vi "Daj Boze nesto.vi"() -> ()   [LabVIEW 2014]
uses:
  Timer 2013/Control Timer.ctl
  <vilib>/ptbypt/NI_PtbyPt.lvlib
panel:
  in  "Emergency offAct":bool=TRUE
  in  "RightAct":bool
  in  "CenterAct":bool
  in  "LeftAct":bool
  in  "OffAct":bool=TRUE
  in  "OnAct":bool
  out "PumpFlag":bool
  out "SDFlag":bool
  out "error out":errorcluster
  in  "error in (no error)":errorcluster
  in  "Center":bool
  in  "Left":bool
  in  "Right":bool
  in  "Emergency off":bool=TRUE
  in  "Off":bool=TRUE
  in  "On":bool
  out "Stanje":string
  out "RightLED":bool
  out "LeftLED":bool
  out "CenterLED":bool
  out "Fault":bool
  out "On/Off":bool
  out "BrojacGreska":dbl
  out "Brojac":dbl
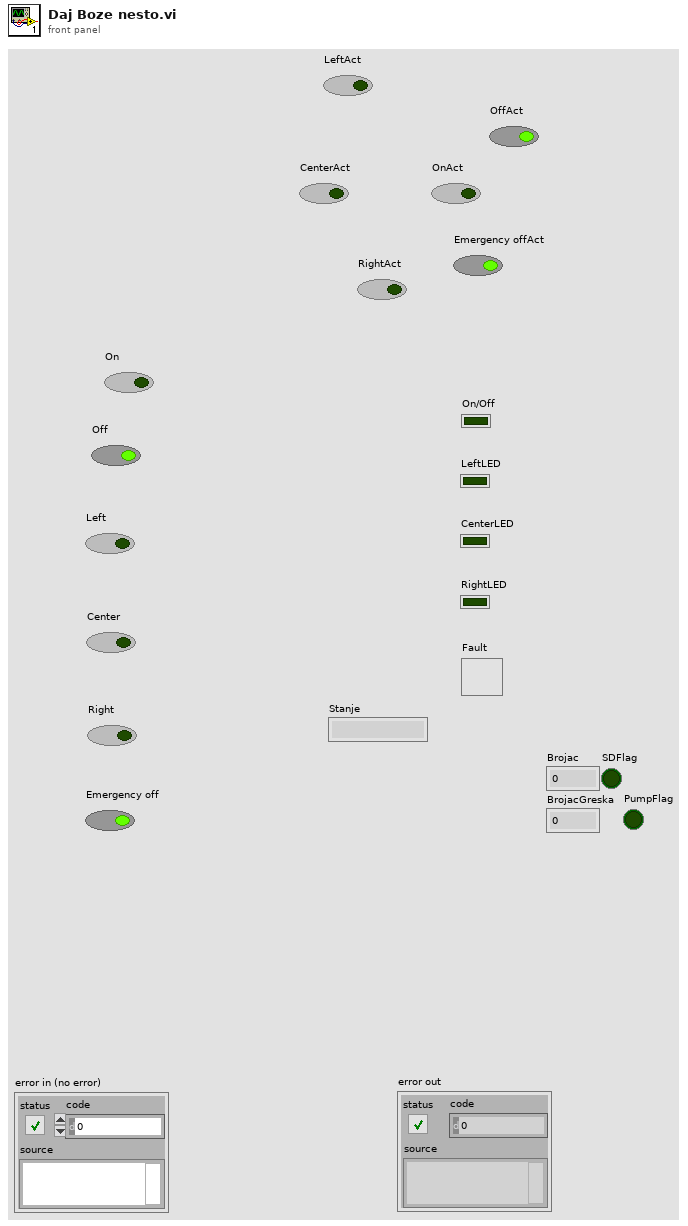
[diagram p1: front panel]
types:
  T1 = typedef "Control Timer.ctl" = enum16{"Timecheck", "Reset"}
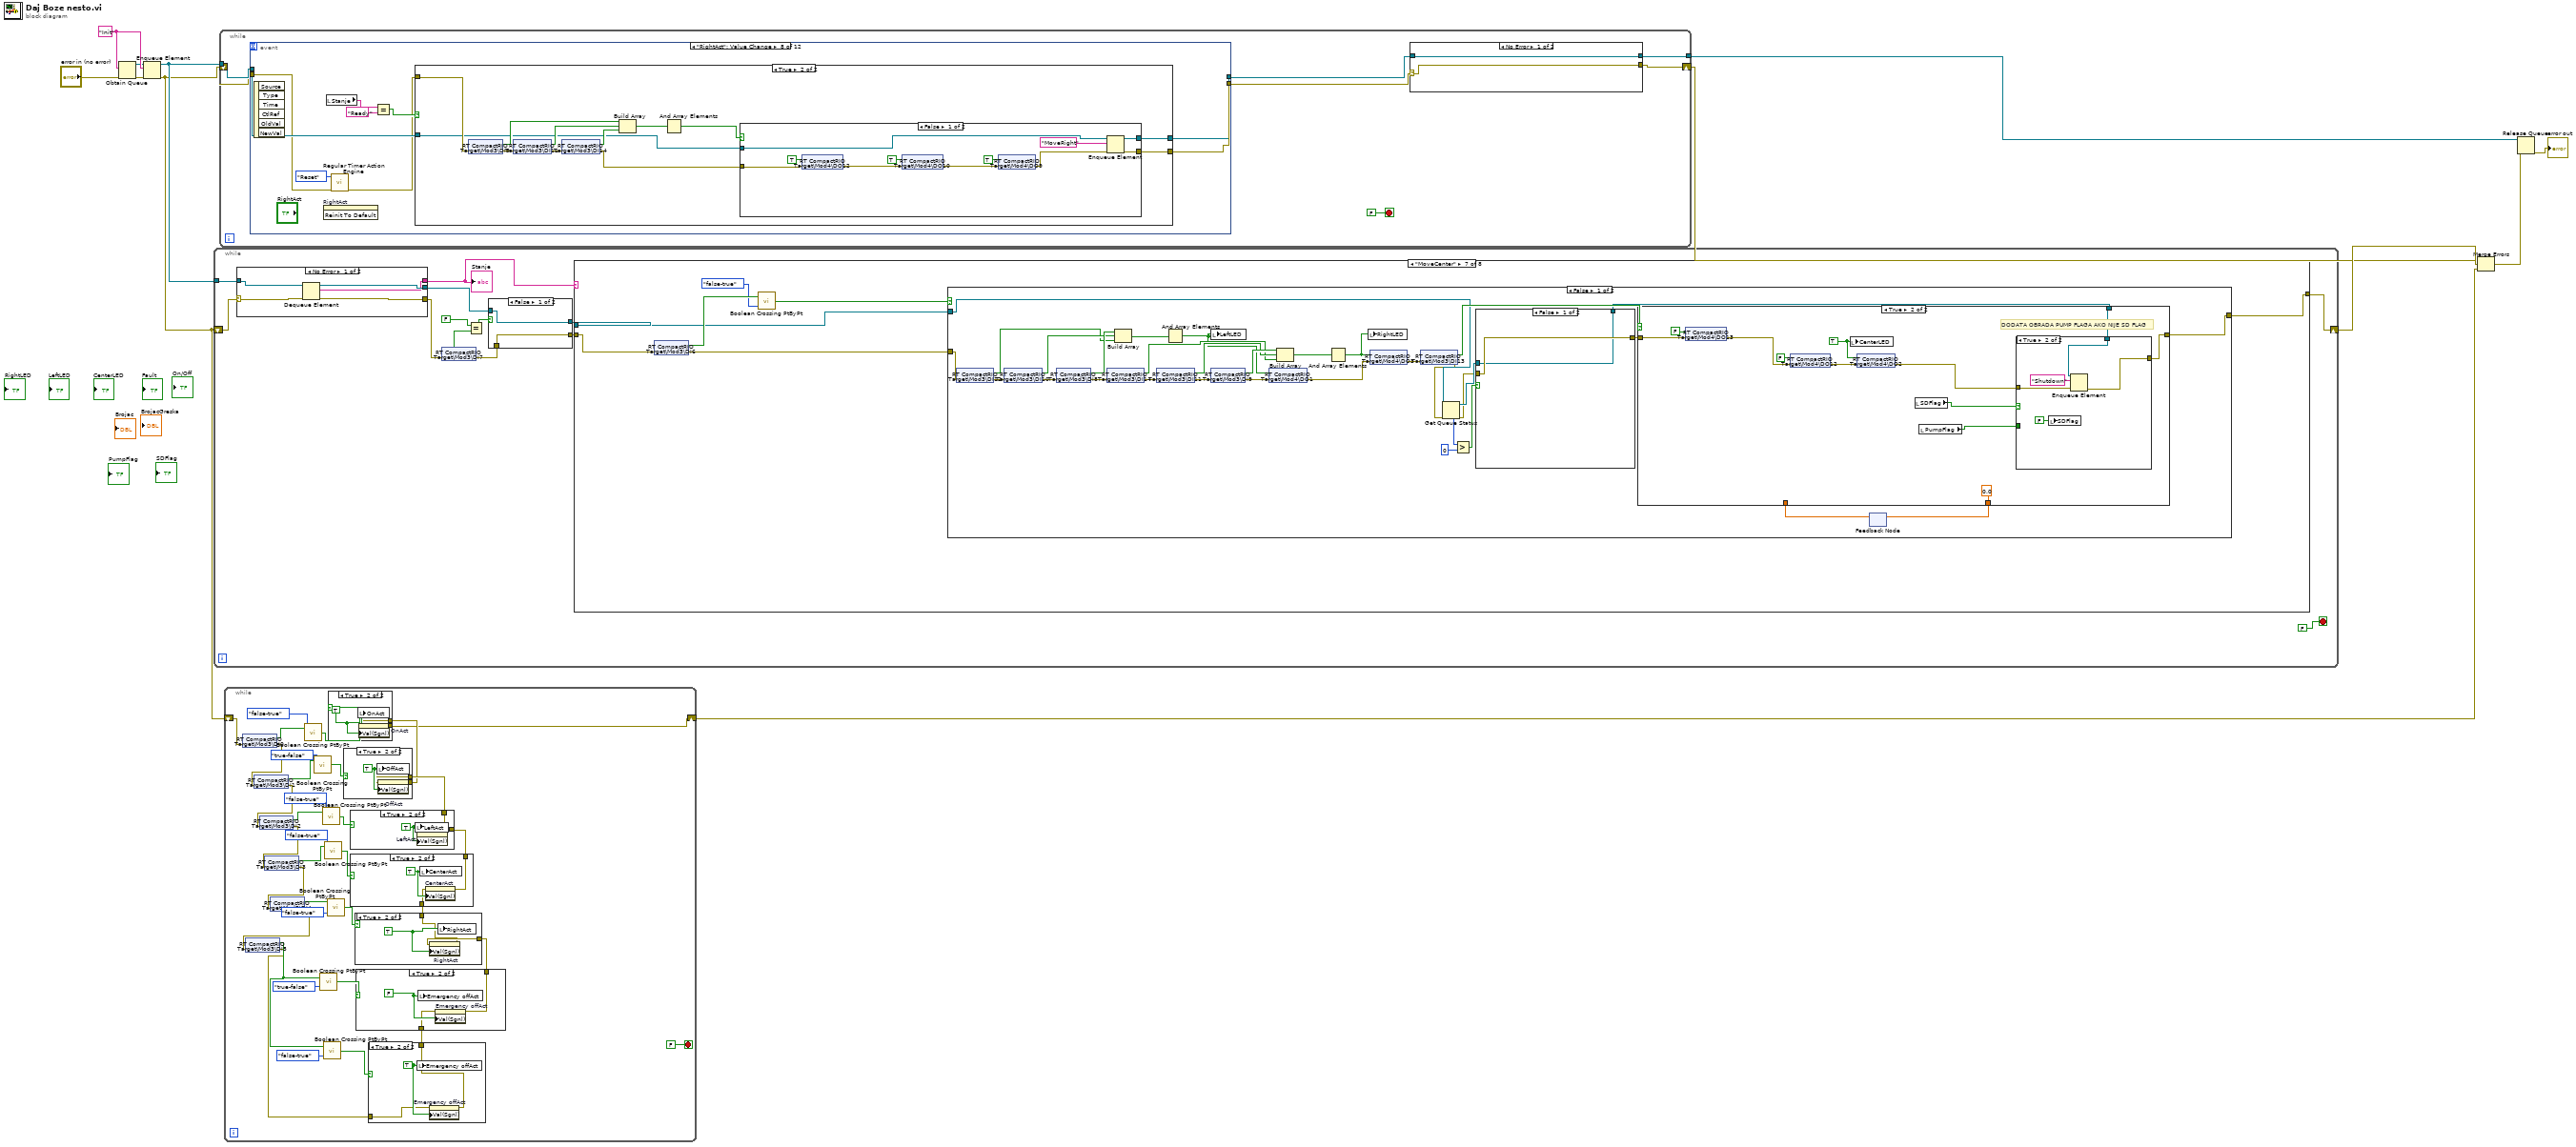
[diagram p0: block diagram]
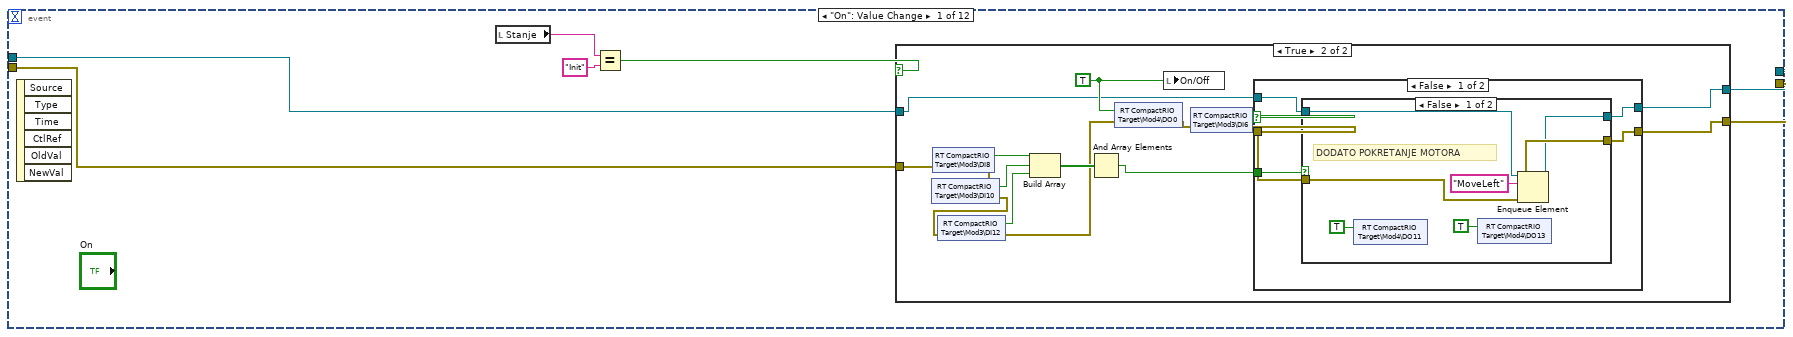
[diagram p9: hidden frame]
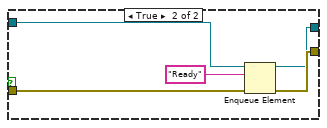
[diagram p11: hidden frame]
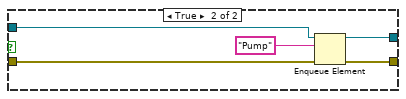
[diagram p12: hidden frame]
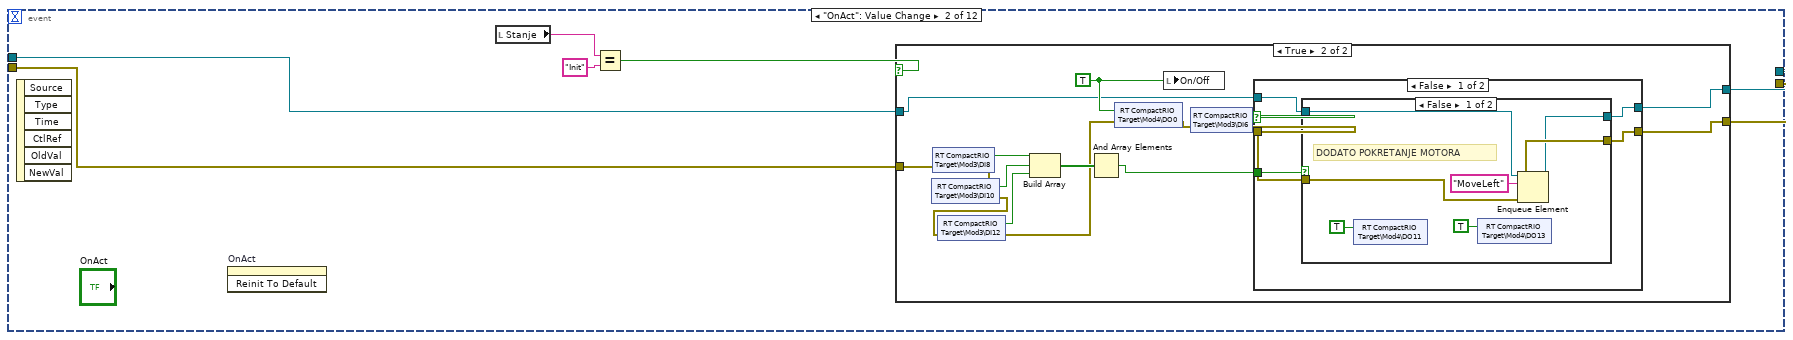
[diagram p13: hidden frame]
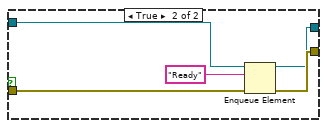
[diagram p15: hidden frame]
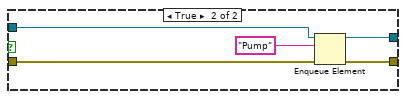
[diagram p16: hidden frame]
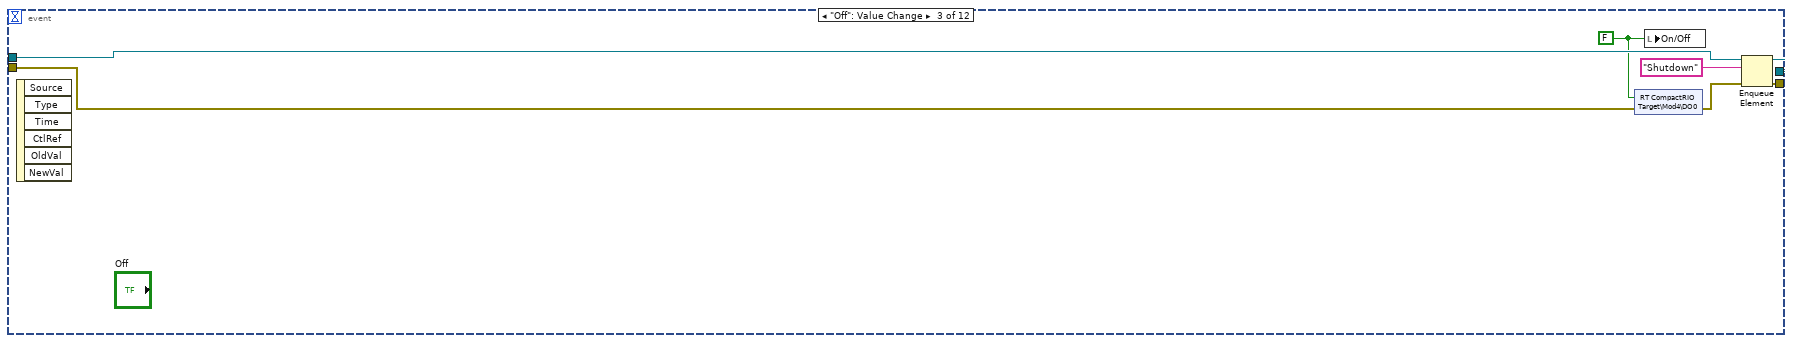
[diagram p17: hidden frame]
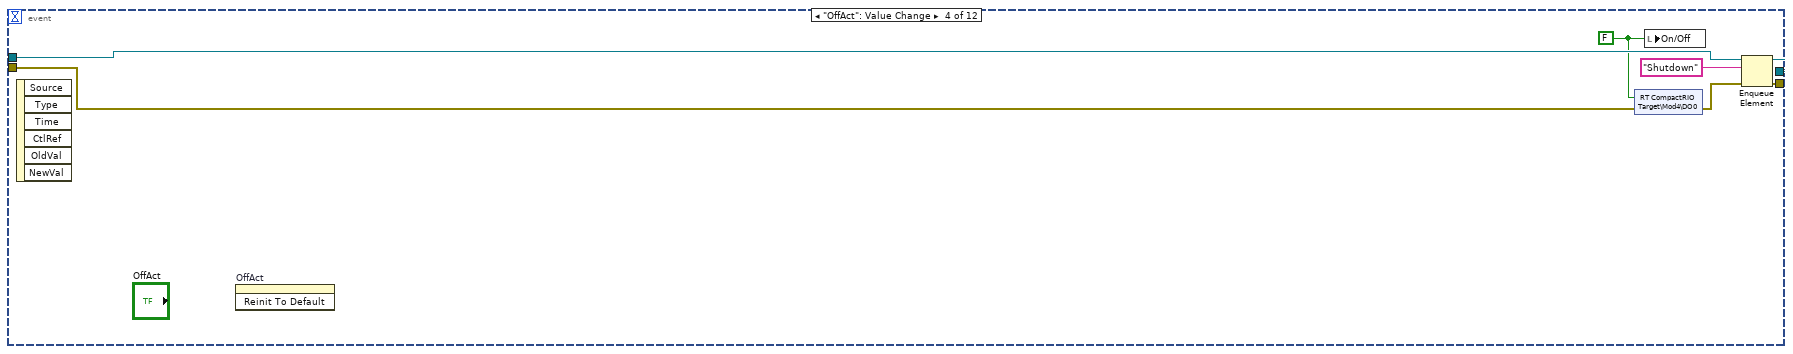
[diagram p18: hidden frame]
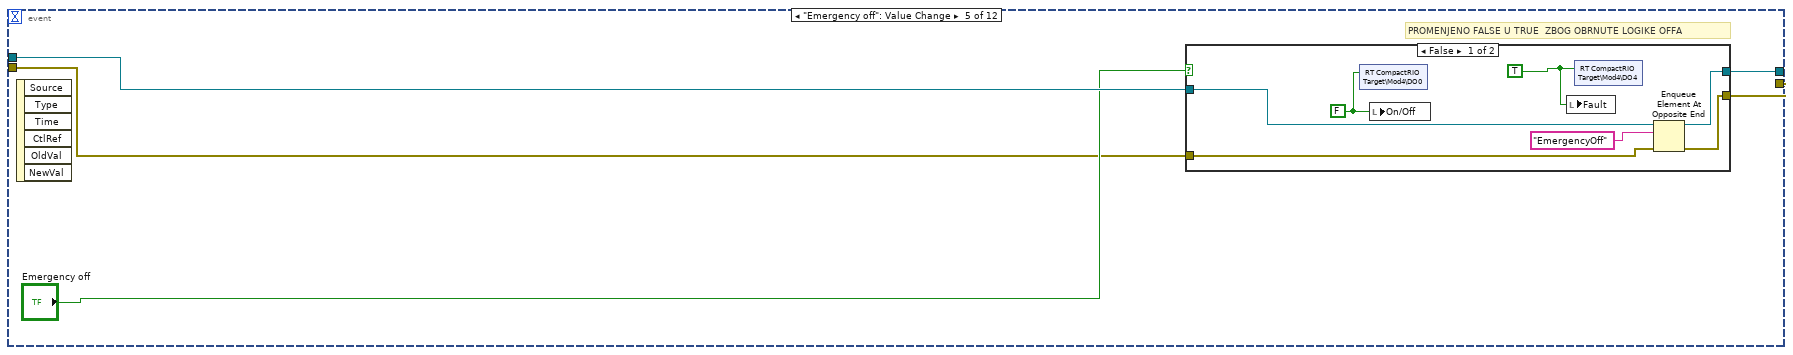
[diagram p19: hidden frame]
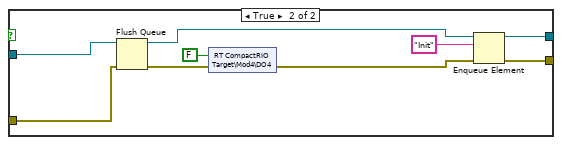
[diagram p20: hidden frame]
diagram:
  w12 = "Init"
  n1 = Obtain Queue(element data type=w12, error in (no error)="error in (no error)") -> (queue out=w10:refnum<queue>, error out=w11:errorcluster)  [unwired: 3 in, 1 out]
  n2 = Enqueue Element(queue=w10, element=w12, error in (no error)=w11) -> (queue out=w9:refnum<queue>, error out=w2:errorcluster)  [unwired: 1 in, 1 out]
  n3 = while {
    tunnel: w9 -> [w25]
    shift-right: [w13] -> w6
    shift-left: w2 -> [w14]
    stop <- FALSE stop-if-true
    n4 = case shown="No Error" w14 {
      selector: w14 -> [w686 w691]
      tunnel: w25 -> [w682 w690]
      tunnel: [w685 w689] -> w23
      tunnel: [w684 w688] -> w17
      tunnel: [w683 w687] -> w24
      frame No Error {
        n5 = Dequeue Element(queue=w682, error in (no error)=w686) -> (queue out=w684:refnum<queue>, element=w683:string, error out=w685:errorcluster)  [unwired: 1 in, 1 out]
      }
      frame Error {
        w687 = "Shutdown" ("element")
        n6 = Enqueue Element(queue=w690, element=w687, error in (no error)=w691) -> (queue out=w688:refnum<queue>, error out=w689:errorcluster)  [unwired: 1 in, 1 out]
      }
    }
    "Stanje" <- w24
    n7 = shared-variable "RT CompactRIO Target\\Mod3\\DI7"(error in=w23) -> (w22:bool, error out=w19:errorcluster)
    n8 = Equal?(x=FALSE, y=w22) -> (x = y?=w20:bool)
    n9 = case shown="False" w20 {
      tunnel: w19 -> [w27 w29]
      tunnel: [w27 w31] -> w18
      tunnel: w17 -> [w26 w28]
      tunnel: [w26 w30] -> w16
      frame False {
      }
      frame True {
        n10 = Enqueue Element At Opposite End(queue=w28, element="EmergencyOff", error in (no error)=w29) -> (queue out=w30:refnum<queue>, error out=w31:errorcluster)  [unwired: 1 in, 1 out]
      }
    }
    n11 = case shown="\"MoveCenter\"" w24 {
      selector: w24 -> [_ _ _ _ _ _ _ w637]
      tunnel: [w44 w83 w104 w144 w198 w351 w503 w638] -> w13
      tunnel: w18 -> [w39 w87 w105 w143 w192 w345 w497 w634]
      tunnel: w16 -> [_ w82 w102 w140 w193 w346 w498 w636]
      frame "Init", Default {
        # "DOADATA REINIICILIZACIJA NOVIH PROMENLJIVIH"
        n12 = shared-variable "RT CompactRIO Target\\Mod4\\DO0"(FALSE ("DO0"), error in=w39) -> (error out=w38:errorcluster)
        n13 = shared-variable "RT CompactRIO Target\\Mod3\\DI12"(error in=w38) -> (w73:bool, error out=w71:errorcluster)
        n14 = shared-variable "RT CompactRIO Target\\Mod3\\DI10"(error in=w71) -> (w74:bool, error out=w70:errorcluster)
        n15 = shared-variable "RT CompactRIO Target\\Mod3\\DI8"(error in=w70) -> (w75:bool, error out=w60:errorcluster)
        n16 = Build Array(w75, w74, w73) -> (w72:bool[])
        n17 = And Array Elements(Boolean array=w72) -> (logical AND=w56:bool)
        n18 = local write "LeftLED"(w56) -> ()
        n19 = shared-variable "RT CompactRIO Target\\Mod4\\DO1"(w56, error in=w60) -> (error out=w59:errorcluster)
        n20 = shared-variable "RT CompactRIO Target\\Mod3\\DI14"(error in=w59) -> (w67:bool, error out=w65:errorcluster)
        n21 = shared-variable "RT CompactRIO Target\\Mod3\\DI11"(error in=w65) -> (w68:bool, error out=w64:errorcluster)
        n22 = shared-variable "RT CompactRIO Target\\Mod3\\DI9"(error in=w64) -> (w69:bool, error out=w58:errorcluster)
        n23 = Build Array(w69, w68, w67) -> (w66:bool[])
        n24 = And Array Elements(Boolean array=w66) -> (logical AND=w54:bool)
        n25 = local write "RightLED"(w54) -> ()
        n26 = shared-variable "RT CompactRIO Target\\Mod4\\DO3"(w54, error in=w58) -> (error out=w57:errorcluster)
        n27 = shared-variable "RT CompactRIO Target\\Mod3\\DI13"(error in=w57) -> (w55:bool, error out=w63:errorcluster)
        n28 = local write "Fault"(FALSE) -> ()
        n29 = local write "CenterLED"(w55) -> ()
        n30 = shared-variable "RT CompactRIO Target\\Mod4\\DO2"(w55, error in=w63) -> (error out=w52:errorcluster)
        n31 = shared-variable "RT CompactRIO Target\\Mod4\\DO4"(FALSE ("DO4"), error in=w52) -> (error out=w51:errorcluster)
        n32 = shared-variable "RT CompactRIO Target\\Mod4\\DO13"(FALSE ("DO15"), error in=w51) -> (error out=w37:errorcluster)
        n33 = shared-variable "RT CompactRIO Target\\Mod4\\DO12"(FALSE ("DO14"), error in=w37) -> (error out=w62:errorcluster)
        n34 = shared-variable "RT CompactRIO Target\\Mod4\\DO11"(FALSE ("DO13"), error in=w62) -> (error out=w43:errorcluster)
        n35 = shared-variable "RT CompactRIO Target\\Mod4\\DO8"(FALSE ("DO10"), error in=w43) -> (error out=w42:errorcluster)
        n36 = shared-variable "RT CompactRIO Target\\Mod4\\DO10"(FALSE ("DO12"), error in=w42) -> (error out=w61:errorcluster)
        n37 = shared-variable "RT CompactRIO Target\\Mod4\\DO9"(FALSE ("DO11"), error in=w61) -> (error out=w35:errorcluster)
        n38 = invoke on="SDFlag" class="Bool (strict)" method="Reinit To Default"(error in=w35) -> (error out=w34:errorcluster)  [unwired: 2 in, 2 out]
        n39 = invoke on="PumpFlag" class="Bool (strict)" method="Reinit To Default"(error in=w34) -> (error out=w33:errorcluster)  [unwired: 2 in, 2 out]
        n40 = invoke on="On/Off" class="Bool (strict)" method="Reinit To Default"(error in=w33) -> (error out=w41:errorcluster)  [unwired: 2 in, 2 out]
        n41 = invoke on="On" class="Bool" method="Reinit To Default"(error in=w41) -> (error out=w45:errorcluster)  [unwired: 2 in, 2 out]
        n42 = invoke on="Off" class="Bool" method="Reinit To Default"(error in=w45) -> (error out=w49:errorcluster)  [unwired: 2 in, 2 out]
        n43 = invoke on="Emergency off" class="Bool (strict)" method="Reinit To Default"(error in=w49) -> (error out=w48:errorcluster)  [unwired: 2 in, 2 out]
        n44 = invoke on="Right" class="Bool" method="Reinit To Default"(error in=w48) -> (error out=w47:errorcluster)  [unwired: 2 in, 2 out]
        n45 = invoke on="Left" class="Bool" method="Reinit To Default"(error in=w47) -> (error out=w46:errorcluster)  [unwired: 2 in, 2 out]
        n46 = invoke on="Center" class="Bool" method="Reinit To Default"(error in=w46) -> (error out=w44:errorcluster)  [unwired: 2 in, 2 out]
      }
      frame "Shutdown" {
        n47 = shared-variable "RT CompactRIO Target\\Mod4\\DO8"(FALSE ("DO8"), error in=w87) -> (error out=w86:errorcluster)
        n48 = shared-variable "RT CompactRIO Target\\Mod4\\DO9"(FALSE ("DO11"), error in=w86) -> (error out=w96:errorcluster)
        n49 = shared-variable "RT CompactRIO Target\\Mod4\\DO10"(FALSE ("DO12"), error in=w96) -> (error out=w88:errorcluster)
        n50 = shared-variable "RT CompactRIO Target\\Mod4\\DO11"(FALSE ("DO13"), error in=w88) -> (error out=w95:errorcluster)
        n51 = shared-variable "RT CompactRIO Target\\Mod4\\DO12"(FALSE ("DO14"), error in=w95) -> (error out=w94:errorcluster)
        n52 = shared-variable "RT CompactRIO Target\\Mod4\\DO13"(FALSE ("DO15"), error in=w94) -> (error out=w84:errorcluster)
        n53 = Enqueue Element(queue=w82, element="Init", error in (no error)=w84) -> (error out=w83:errorcluster)  [unwired: 1 in, 2 out]
      }
      frame "EmergencyOff" {
        w108 = TRUE ("DO4")
        n54 = shared-variable "RT CompactRIO Target\\Mod4\\DO12"(FALSE ("DO14"), error in=w105) -> (error out=w110:errorcluster)
        n55 = shared-variable "RT CompactRIO Target\\Mod4\\DO4"(w108, error in=w110) -> (error out=w109:errorcluster)
        n56 = local write "Fault"(w108) -> ()
        n57 = shared-variable "RT CompactRIO Target\\Mod4\\DO13"(FALSE ("DO15"), error in=w109) -> (error out=w112:errorcluster)
        n58 = shared-variable "RT CompactRIO Target\\Mod4\\DO9"(FALSE ("DO11"), error in=w112) -> (error out=w118:errorcluster)
        n59 = shared-variable "RT CompactRIO Target\\Mod4\\DO10"(FALSE ("DO12"), error in=w118) -> (error out=w111:errorcluster)
        n60 = shared-variable "RT CompactRIO Target\\Mod4\\DO11"(FALSE ("DO13"), error in=w111) -> (error out=w107:errorcluster)
        n61 = shared-variable "RT CompactRIO Target\\Mod4\\DO8"(FALSE ("DO8"), error in=w107) -> (error out=w101:errorcluster)
        n62 = Get Queue Status(queue=w102, error in (no error)=w101) -> (queue out=w103:refnum<queue>, error out=w100:errorcluster, # elements in queue=w99:i32)  [unwired: 1 in, 5 out]
        n63 = Greater?(x=w99, y=0) -> (0:w97:bool)
        n64 = case shown="False" w97 {
          tunnel: [w119 w125] -> w104
          tunnel: w103 -> [w121 w124]
          tunnel: w100 -> [w120 w123]
          frame False {
            n65 = Enqueue Element At Opposite End(queue=w121, element="EmergencyOff", error in (no error)=w120) -> (error out=w119:errorcluster)  [unwired: 1 in, 2 out]
          }
          frame True {
            # "DODATA PROVERA DA LI SE POJAVIO INIT TJ DA LI JE UGASEN EM OFF DA GA NE BISMO VISE DODAVALI"
            n66 = Preview Queue Element(queue=w124, error in (no error)=w123) -> (queue out=w128:refnum<queue>, element=w130:string, error out=w127:errorcluster)  [unwired: 1 in, 1 out]
            n67 = Equal?(x=w130, y="Init") -> (x = y?=w126:bool)
            n68 = case shown="False" w126 {
              tunnel: w128 -> [w133 _]
              tunnel: w127 -> [w132 w135]
              tunnel: [w131 w135] -> w125
              frame False {
                n69 = Enqueue Element At Opposite End(queue=w133, element="EmergencyOff", error in (no error)=w132) -> (error out=w131:errorcluster)  [unwired: 1 in, 2 out]
              }
              frame True {
              }
            }
          }
        }
      }
      frame "Pump" {
        n70 = shared-variable "RT CompactRIO Target\\Mod3\\DI6"(error in=w143) -> (w146:bool, error out=w142:errorcluster)
        n71 = call <vilib>:"Boolean Crossing PtByPt.vi"("direction"=enum16{"either", "false-true", "true-false"}."true-false", "input"=w146) -> ("crossing"=w145:bool)  [unwired: 1 in]
        n72 = Get Queue Status(queue=w140, error in (no error)=w142) -> (queue out=w139:refnum<queue>, error out=w141:errorcluster, # elements in queue=w138:i32)  [unwired: 1 in, 5 out]
        n73 = Greater?(x=w138, y=0) -> (0:w136:bool)
        n74 = case shown="True" w136 {
          tunnel: w145 -> [w151 w172]
          tunnel: [w149 w171] -> w144
          tunnel: w141 -> [w150 w168]
          tunnel: w139 -> [w148 w170]
          frame False {
            n75 = case shown="True" w151 {
              tunnel: w150 -> [w153 w159]
              tunnel: [w156 w162] -> w149
              tunnel: w148 -> [w155 w161]
              frame False {
                n76 = shared-variable "RT CompactRIO Target\\Mod4\\DO8"(TRUE ("DO8"), error in=w153) -> (error out=w152:errorcluster)
                n77 = Enqueue Element(queue=w155, element="Pump", error in (no error)=w152) -> (error out=w156:errorcluster)  [unwired: 1 in, 2 out]
              }
              frame True {
                n78 = shared-variable "RT CompactRIO Target\\Mod4\\DO8"(FALSE ("DO8"), error in=w159) -> (error out=w158:errorcluster)
                n79 = Enqueue Element(queue=w161, element="Ready", error in (no error)=w158) -> (error out=w162:errorcluster)  [unwired: 1 in, 2 out]
              }
            }
          }
          frame True {
            n80 = Preview Queue Element(queue=w170, error in (no error)=w168) -> (queue out=w169:refnum<queue>, element=w166:string, error out=w167:errorcluster)  [unwired: 1 in, 1 out]
            n81 = Equal?(x=w166, y="Shutdown") -> (x = y?=w164:bool)
            n82 = case shown="False" w164 {
              tunnel: w172 -> [w176 _]
              tunnel: w167 -> [w175 w190]
              tunnel: [w174 w189] -> w171
              tunnel: w169 -> [w173 _]
              frame False {
                n83 = case shown="True" w176 {
                  tunnel: w175 -> [w179 w185]
                  tunnel: [w182 w188] -> w174
                  tunnel: w173 -> [w177 w183]
                  frame False {
                    n84 = shared-variable "RT CompactRIO Target\\Mod4\\DO8"(TRUE ("DO10"), error in=w179) -> (error out=w178:errorcluster)
                    n85 = Enqueue Element(queue=w177, element="Pump", error in (no error)=w178) -> (error out=w182:errorcluster)  [unwired: 1 in, 2 out]
                  }
                  frame True {
                    n86 = shared-variable "RT CompactRIO Target\\Mod4\\DO8"(FALSE ("DO10"), error in=w185) -> (error out=w184:errorcluster)
                    n87 = Enqueue Element At Opposite End(queue=w183, element="Ready", error in (no error)=w184) -> (error out=w188:errorcluster)  [unwired: 1 in, 2 out]
                  }
                }
              }
              frame True {
                n88 = shared-variable "RT CompactRIO Target\\Mod4\\DO8"(FALSE ("DO8"), error in=w190) -> (error out=w189:errorcluster)
              }
            }
          }
        }
      }
      frame "MoveRight" {
        n89 = shared-variable "RT CompactRIO Target\\Mod3\\DI6"(error in=w192) -> (w196:bool, error out=w197:errorcluster)
        n90 = call <vilib>:"Boolean Crossing PtByPt.vi"("direction"=enum16{"either", "false-true", "true-false"}."false-true", "input"=w196) -> ("crossing"=w194:bool)  [unwired: 1 in]
        n91 = case shown="False" w194 {
          tunnel: w197 -> [w230 w343]
          tunnel: [w227 w342] -> w198
          tunnel: w193 -> [w204 w340]
          frame False {
            n92 = shared-variable "RT CompactRIO Target\\Mod3\\DI9"(error in=w230) -> (w234:bool, error out=w229:errorcluster)
            n93 = shared-variable "RT CompactRIO Target\\Mod3\\DI11"(error in=w229) -> (w233:bool, error out=w228:errorcluster)
            n94 = shared-variable "RT CompactRIO Target\\Mod3\\DI14"(error in=w228) -> (w232:bool, error out=w216:errorcluster)
            n95 = shared-variable "RT CompactRIO Target\\Mod3\\DI12"(error in=w216) -> (w223:bool, error out=w221:errorcluster)
            n96 = Build Array(w234, w233, w232) -> (w231:bool[])
            n97 = shared-variable "RT CompactRIO Target\\Mod3\\DI10"(error in=w221) -> (w224:bool, error out=w220:errorcluster)
            n98 = And Array Elements(Boolean array=w231) -> (logical AND=w226:bool)
            n99 = shared-variable "RT CompactRIO Target\\Mod3\\DI8"(error in=w220) -> (w225:bool, error out=w219:errorcluster)
            n100 = shared-variable "RT CompactRIO Target\\Mod3\\DI13"(error in=w219) -> (w214:bool, error out=w218:errorcluster)
            n101 = Build Array(w225, w224, w223) -> (w222:bool[])
            n102 = local write "CenterLED"(w214) -> ()
            n103 = shared-variable "RT CompactRIO Target\\Mod4\\DO2"(w214, error in=w218) -> (error out=w217:errorcluster)
            n104 = And Array Elements(Boolean array=w222) -> (logical AND=w215:bool)
            n105 = shared-variable "RT CompactRIO Target\\Mod4\\DO1"(w215, error in=w217) -> (error out=w205:errorcluster)
            n106 = Get Queue Status(queue=w204, error in (no error)=w205) -> (queue out=w202:refnum<queue>, error out=w203:errorcluster, # elements in queue=w201:i32)  [unwired: 1 in, 5 out]
            n107 = local write "LeftLED"(w215) -> ()
            n108 = Greater?(x=w201, y=0) -> (0:w199:bool)
            n109 = case shown="True" w199 {
              tunnel: w202 -> [w236 w245]
              tunnel: w203 -> [w235 w244]
              tunnel: [w236 w241] -> w209
              tunnel: [w235 w240] -> w208
              frame False {
              }
              frame True {
                n110 = Preview Queue Element(queue=w245, error in (no error)=w244) -> (queue out=w242:refnum<queue>, element=w238:string, error out=w243:errorcluster)  [unwired: 1 in, 1 out]
                n111 = Equal?(x=w238, y="Shutdown") -> (x = y?=w239:bool)
                n112 = case shown="True" w239 {
                  tunnel: w243 -> [w246 w251]
                  tunnel: w242 -> [w247 w250]
                  tunnel: [w247 w249] -> w241
                  tunnel: [w246 w248] -> w240
                  frame False {
                  }
                  frame True {
                    n113 = Flush Queue(queue=w250, error in (no error)=w251) -> (queue out=w249:refnum<queue>, error out=w248:errorcluster)  [unwired: 1 out]
                    n114 = local write "SDFlag"(TRUE ("SDFlag")) -> ()
                  }
                }
              }
            }
            n115 = feedback #1(0.0) -> (w211:dbl)
            n116 = feedback #2(0.0) -> (w213:dbl)
            n117 = case shown="False" w226 {
              tunnel: [w261 w321] -> w227
              tunnel: w213 -> [w258 _]
              tunnel: [w257 0.0] -> w212
              tunnel: w211 -> [w256 _]
              tunnel: [w255 0.0] -> w210
              tunnel: w209 -> [w253 w312]
              tunnel: w208 -> [w254 w311]
              frame False {
                n118 = call "Regular Timer Action Engine.vi"("Enum"=Control_Timer."Timecheck", "Time Target"=0.5, "error in"=w254) -> ("Status"=w267:cluster{"Running":bool, "Done":bool}, "error out"=w264:errorcluster)  [unwired: 6 in]
                n119 = Unbundle By Name(w267) -> ("Done"=w266:bool)  [unwired: 1 out]
                n120 = feedback #3() -> (w265:bool)  [unwired: 1 in]
                n121 = case shown="True" w266 {
                  tunnel: [w275 w294] -> w260
                  tunnel: w265 -> [w275 w293]
                  tunnel: w264 -> [w274 w291]
                  tunnel: [w274 w285] -> w263
                  tunnel: w256 -> [w273 w290]
                  tunnel: [w273 w286] -> w255
                  tunnel: w258 -> [w272 w284]
                  tunnel: [w272 w281] -> w257
                  tunnel: [w271 w280] -> w259
                  tunnel: w253 -> [w271 w276]
                  frame False {
                  }
                  frame True {
                    n122 = Increment(x=w290) -> (x+1=w287:dbl)
                    n123 = Increment(x=w284) -> (x+1=w279:dbl)
                    n124 = local write "Brojac"(w287) -> ()
                    n125 = local write "BrojacGreska"(w279) -> ()
                    n126 = Not(x=w293) -> (.not. x?=w294:bool)
                    n127 = Greater Or Equal?(x=w279, y=29.0) -> (x >= y?=w282:bool)
                    n128 = Greater Or Equal?(x=3.0, y=w287) -> (x >= y?=w289:bool)
                    n129 = call "Regular Timer Action Engine.vi"("Enum"=Control_Timer."Reset", "error in"=w291) -> ("error out"=w278:errorcluster)  [unwired: 7 in, 1 out]
                    n130 = case shown="True" w282 {
                      tunnel: [w297 0.0] -> w281
                      tunnel: w279 -> [w297 _]
                      tunnel: [w295 w301] -> w280
                      tunnel: w278 -> [w296 w298]
                      tunnel: [w296 w300] -> w277
                      tunnel: w276 -> [w295 w299]
                      frame False {
                      }
                      frame True {
                        n131 = Enqueue Element At Opposite End(queue=w299, element="EmergencyOff", error in (no error)=w298) -> (queue out=w301:refnum<queue>, error out=w300:errorcluster)  [unwired: 1 in, 1 out]
                      }
                    }
                    n132 = case shown="True" w289 {
                      tunnel: w287 -> [w305 _]
                      tunnel: [w305 0.0] -> w286
                      tunnel: [w304 w306] -> w285
                      tunnel: w277 -> [w304 w306]
                      frame False {
                      }
                      frame True {
                        n133 = shared-variable "RT CompactRIO Target\\Mod4\\DO10"(FALSE ("DO12")) -> ()  [unwired: 1 in, 1 out]
                      }
                    }
                  }
                }
                n134 = feedback-in #3(w260) -> ()
                n135 = local write "RightLED"(w260) -> ()
                n136 = shared-variable "RT CompactRIO Target\\Mod4\\DO3"(w260, error in=w263) -> (error out=w262:errorcluster)
                n137 = Enqueue Element(queue=w259, element="MoveRight", error in (no error)=w262) -> (error out=w261:errorcluster)  [unwired: 1 in, 2 out]
              }
              frame True {
                w315 = TRUE ("DO3")
                # "DODATA OBRADA PUMP FLAGA AKO NIJE SD FLAG"
                n138 = shared-variable "RT CompactRIO Target\\Mod4\\DO12"(FALSE ("DO15"), error in=w311) -> (error out=w318:errorcluster)
                n139 = shared-variable "RT CompactRIO Target\\Mod4\\DO10"(FALSE ("DO13"), error in=w318) -> (error out=w317:errorcluster)
                n140 = local write "RightLED"(w315) -> ()
                n141 = shared-variable "RT CompactRIO Target\\Mod4\\DO3"(w315, error in=w317) -> (error out=w316:errorcluster)
                n142 = local read "SDFlag"() -> (w310:bool)
                n143 = local read "PumpFlag"() -> (w309:bool)
                n144 = case shown="True" w310 {
                  tunnel: [w325 w339] -> w321
                  tunnel: w316 -> [w324 w335]
                  tunnel: w312 -> [w323 w336]
                  tunnel: w309 -> [w322 _]
                  frame False {
                    n145 = case shown="True" w322 {
                      tunnel: [w328 w332] -> w325
                      tunnel: w324 -> [w327 w333]
                      tunnel: w323 -> [w326 w334]
                      frame False {
                        n146 = Enqueue Element(queue=w326, element="Ready", error in (no error)=w327) -> (error out=w328:errorcluster)  [unwired: 1 in, 2 out]
                      }
                      frame True {
                        n147 = local write "PumpFlag"(FALSE ("PumpFlag")) -> ()
                        n148 = Enqueue Element(queue=w334, element="Pump", error in (no error)=w333) -> (error out=w332:errorcluster)  [unwired: 1 in, 2 out]
                      }
                    }
                  }
                  frame True {
                    n149 = local write "SDFlag"(FALSE ("SDFlag")) -> ()
                    n150 = Enqueue Element(queue=w336, element="Shutdown", error in (no error)=w335) -> (error out=w339:errorcluster)  [unwired: 1 in, 2 out]
                  }
                }
              }
            }
            n151 = feedback-in #1(w210) -> ()
            n152 = feedback-in #2(w212) -> ()
          }
          frame True {
            # "DODAT FALG UMESTO POKRETANJA PUMPE ODMAH"
            n153 = local write "PumpFlag"(TRUE ("PumpFlag")) -> ()
            n154 = Enqueue Element(queue=w340, element="MoveRight", error in (no error)=w343) -> (error out=w342:errorcluster)  [unwired: 1 in, 2 out]
          }
        }
      }
      frame "MoveLeft" {
        n155 = shared-variable "RT CompactRIO Target\\Mod3\\DI6"(error in=w345) -> (w350:bool, error out=w348:errorcluster)
        n156 = call <vilib>:"Boolean Crossing PtByPt.vi"("direction"=enum16{"either", "false-true", "true-false"}."false-true", "input"=w350) -> ("crossing"=w347:bool)  [unwired: 1 in]
        n157 = case shown="False" w347 {
          tunnel: w348 -> [w380 w494]
          tunnel: [w377 w493] -> w351
          tunnel: w346 -> [w358 w492]
          frame False {
            n158 = shared-variable "RT CompactRIO Target\\Mod3\\DI8"(error in=w380) -> (w385:bool, error out=w379:errorcluster)
            n159 = shared-variable "RT CompactRIO Target\\Mod3\\DI10"(error in=w379) -> (w384:bool, error out=w378:errorcluster)
            n160 = shared-variable "RT CompactRIO Target\\Mod3\\DI12"(error in=w378) -> (w383:bool, error out=w372:errorcluster)
            n161 = shared-variable "RT CompactRIO Target\\Mod3\\DI14"(error in=w372) -> (w374:bool, error out=w371:errorcluster)
            n162 = Build Array(w385, w384, w383) -> (w382:bool[])
            n163 = shared-variable "RT CompactRIO Target\\Mod3\\DI11"(error in=w371) -> (w375:bool, error out=w370:errorcluster)
            n164 = And Array Elements(Boolean array=w382) -> (logical AND=w381:bool)
            n165 = shared-variable "RT CompactRIO Target\\Mod3\\DI9"(error in=w370) -> (w376:bool, error out=w369:errorcluster)
            n166 = shared-variable "RT CompactRIO Target\\Mod3\\DI13"(error in=w369) -> (w365:bool, error out=w368:errorcluster)
            n167 = Build Array(w376, w375, w374) -> (w373:bool[])
            n168 = local write "CenterLED"(w365) -> ()
            n169 = shared-variable "RT CompactRIO Target\\Mod4\\DO2"(w365, error in=w368) -> (error out=w367:errorcluster)
            n170 = And Array Elements(Boolean array=w373) -> (logical AND=w366:bool)
            n171 = local write "RightLED"(w366) -> ()
            n172 = shared-variable "RT CompactRIO Target\\Mod4\\DO3"(w366, error in=w367) -> (error out=w357:errorcluster)
            n173 = Get Queue Status(queue=w358, error in (no error)=w357) -> (queue out=w356:refnum<queue>, error out=w355:errorcluster, # elements in queue=w354:i32)  [unwired: 1 in, 5 out]
            n174 = Greater?(x=w354, y=0) -> (0:w352:bool)
            n175 = case shown="False" w352 {
              tunnel: [w386 w391] -> w360
              tunnel: [w387 w390] -> w359
              tunnel: w356 -> [w387 w389]
              tunnel: w355 -> [w386 w388]
              frame False {
              }
              frame True {
                n176 = Preview Queue Element(queue=w389, error in (no error)=w388) -> (queue out=w393:refnum<queue>, element=w396:string, error out=w392:errorcluster)  [unwired: 1 in, 1 out]
                n177 = Equal?(x=w396, y="Shutdown") -> (x = y?=w394:bool)
                n178 = case shown="True" w394 {
                  tunnel: w393 -> [w397 w403]
                  tunnel: w392 -> [w398 w402]
                  tunnel: [w398 w401] -> w391
                  tunnel: [w397 w399] -> w390
                  frame False {
                  }
                  frame True {
                    n179 = Flush Queue(queue=w403, error in (no error)=w402) -> (queue out=w399:refnum<queue>, error out=w401:errorcluster)  [unwired: 1 out]
                    n180 = local write "SDFlag"(TRUE ("SDFlag")) -> ()
                  }
                }
              }
            }
            n181 = feedback #4() -> (w364:dbl)  [unwired: 1 in]
            n182 = feedback #5() -> (w362:dbl)  [unwired: 1 in]
            n183 = case shown="False" w381 {
              tunnel: w360 -> [w408 w469]
              tunnel: [w421 w473] -> w377
              tunnel: w359 -> [w411 w465]
              tunnel: w364 -> [w407 _]
              tunnel: [w406 0.0] -> w363
              tunnel: w362 -> [w405 _]
              tunnel: [w404 0.0] -> w361
              frame False {
                n184 = call "Regular Timer Action Engine.vi"("Enum"=Control_Timer."Timecheck", "Time Target"=0.5, "error in"=w408) -> ("Status"=w417:cluster{"Running":bool, "Done":bool}, "error out"=w414:errorcluster)  [unwired: 6 in]
                n185 = Unbundle By Name(w417) -> ("Done"=w416:bool)  [unwired: 1 out]
                n186 = feedback #6() -> (w415:bool)  [unwired: 1 in]
                n187 = case shown="True" w416 {
                  tunnel: [w426 w445] -> w412
                  tunnel: w415 -> [w426 w444]
                  tunnel: w414 -> [w425 w433]
                  tunnel: [w425 w442] -> w409
                  tunnel: [w424 w438] -> w404
                  tunnel: w405 -> [w424 w441]
                  tunnel: w407 -> [w423 w429]
                  tunnel: w411 -> [w422 w435]
                  tunnel: [w422 w434] -> w410
                  tunnel: [w423 w430] -> w406
                  frame False {
                  }
                  frame True {
                    n188 = Increment(x=w441) -> (x+1=w428:dbl)
                    n189 = local write "Brojac"(w428) -> ()
                    n190 = Increment(x=w429) -> (x+1=w427:dbl)
                    n191 = local write "BrojacGreska"(w427) -> ()
                    n192 = Greater Or Equal?(x=w427, y=29.0) -> (x >= y?=w436:bool)
                    n193 = Greater Or Equal?(x=w428, y=3.0) -> (x >= y?=w439:bool)
                    n194 = Not(x=w444) -> (.not. x?=w445:bool)
                    n195 = case shown="True" w439 {
                      tunnel: w428 -> [w456 _]
                      tunnel: [w456 0.0] -> w438
                      tunnel: w433 -> [w455 w458]
                      tunnel: [w455 w457] -> w432
                      frame False {
                      }
                      frame True {
                        n196 = shared-variable "RT CompactRIO Target\\Mod4\\DO11"(FALSE ("DO13"), error in=w458) -> (error out=w457:errorcluster)
                      }
                    }
                    n197 = case shown="True" w436 {
                      tunnel: w427 -> [w448 _]
                      tunnel: [w448 0.0] -> w430
                      tunnel: w435 -> [w447 w449]
                      tunnel: [w447 w453] -> w434
                      tunnel: w432 -> [w446 w450]
                      tunnel: [w446 w452] -> w431
                      frame False {
                      }
                      frame True {
                        n198 = Enqueue Element At Opposite End(queue=w449, element="EmergencyOff", error in (no error)=w450) -> (queue out=w453:refnum<queue>, error out=w452:errorcluster)  [unwired: 1 in, 1 out]
                      }
                    }
                    n199 = call "Regular Timer Action Engine.vi"("Enum"=Control_Timer."Reset", "error in"=w431) -> ("error out"=w442:errorcluster)  [unwired: 7 in, 1 out]
                  }
                }
                n200 = feedback-in #6(w412) -> ()
                n201 = local write "LeftLED"(w412) -> ()
                n202 = shared-variable "RT CompactRIO Target\\Mod4\\DO1"(w412, error in=w409) -> (error out=w413:errorcluster)
                n203 = Enqueue Element(queue=w410, element="MoveLeft", error in (no error)=w413) -> (error out=w421:errorcluster)  [unwired: 1 in, 2 out]
              }
              frame True {
                w467 = TRUE ("DO1")
                # "DODATA OBRADA PUMP FLAGA AKO NIJE SD FLAG"
                n204 = local write "LeftLED"(w467) -> ()
                n205 = shared-variable "RT CompactRIO Target\\Mod4\\DO1"(w467, error in=w469) -> (error out=w468:errorcluster)
                n206 = shared-variable "RT CompactRIO Target\\Mod4\\DO13"(FALSE ("DO15"), error in=w468) -> (error out=w470:errorcluster)
                n207 = local read "SDFlag"() -> (w462:bool)
                n208 = local read "PumpFlag"() -> (w461:bool)
                n209 = shared-variable "RT CompactRIO Target\\Mod4\\DO11"(FALSE ("DO13"), error in=w470) -> (error out=w466:errorcluster)
                n210 = case shown="True" w462 {
                  tunnel: [w477 w489] -> w473
                  tunnel: w466 -> [w476 w491]
                  tunnel: w465 -> [w475 w490]
                  tunnel: w461 -> [w474 _]
                  frame False {
                    n211 = case shown="True" w474 {
                      tunnel: [w480 w484] -> w477
                      tunnel: w476 -> [w479 w486]
                      tunnel: w475 -> [w478 w485]
                      frame False {
                        n212 = Enqueue Element(queue=w478, element="Ready", error in (no error)=w479) -> (error out=w480:errorcluster)  [unwired: 1 in, 2 out]
                      }
                      frame True {
                        n213 = local write "PumpFlag"(FALSE ("PumpFlag")) -> ()
                        n214 = Enqueue Element(queue=w485, element="Pump", error in (no error)=w486) -> (error out=w484:errorcluster)  [unwired: 1 in, 2 out]
                      }
                    }
                  }
                  frame True {
                    n215 = Enqueue Element(queue=w490, element="Shutdown", error in (no error)=w491) -> (error out=w489:errorcluster)  [unwired: 1 in, 2 out]
                    n216 = local write "SDFlag"(FALSE ("SDFlag")) -> ()
                  }
                }
              }
            }
            n217 = feedback-in #4(w363) -> ()
            n218 = feedback-in #5(w361) -> ()
          }
          frame True {
            # "DODAT FALG UMESTO POKRETANJA PUMPE ODMAH"
            n219 = local write "PumpFlag"(TRUE ("PumpFlag")) -> ()
            n220 = Enqueue Element(queue=w492, element="MoveLeft", error in (no error)=w494) -> (error out=w493:errorcluster)  [unwired: 1 in, 2 out]
          }
        }
      }
      frame "MoveCenter" {
        n221 = shared-variable "RT CompactRIO Target\\Mod3\\DI6"(error in=w497) -> (w502:bool, error out=w499:errorcluster)
        n222 = call <vilib>:"Boolean Crossing PtByPt.vi"("direction"=enum16{"either", "false-true", "true-false"}."false-true", "input"=w502) -> ("crossing"=w500:bool)  [unwired: 1 in]
        n223 = case shown="False" w500 {
          tunnel: [w535 w628] -> w503
          tunnel: w499 -> [w521 w629]
          tunnel: w498 -> [w510 w627]
          frame False {
            n224 = shared-variable "RT CompactRIO Target\\Mod3\\DI12"(error in=w521) -> (w531:bool, error out=w529:errorcluster)
            n225 = shared-variable "RT CompactRIO Target\\Mod3\\DI10"(error in=w529) -> (w532:bool, error out=w528:errorcluster)
            n226 = shared-variable "RT CompactRIO Target\\Mod3\\DI8"(error in=w528) -> (w533:bool, error out=w520:errorcluster)
            n227 = shared-variable "RT CompactRIO Target\\Mod3\\DI14"(error in=w520) -> (w525:bool, error out=w523:errorcluster)
            n228 = Build Array(w533, w532, w531) -> (w530:bool[])
            n229 = shared-variable "RT CompactRIO Target\\Mod3\\DI11"(error in=w523) -> (w526:bool, error out=w522:errorcluster)
            n230 = And Array Elements(Boolean array=w530) -> (logical AND=w515:bool)
            n231 = local write "LeftLED"(w515) -> ()
            n232 = shared-variable "RT CompactRIO Target\\Mod3\\DI9"(error in=w522) -> (w527:bool, error out=w519:errorcluster)
            n233 = shared-variable "RT CompactRIO Target\\Mod4\\DO1"(w515, error in=w519) -> (error out=w518:errorcluster)
            n234 = Build Array(w527, w526, w525) -> (w524:bool[])
            n235 = And Array Elements(Boolean array=w524) -> (logical AND=w516:bool)
            n236 = local write "RightLED"(w516) -> ()
            n237 = shared-variable "RT CompactRIO Target\\Mod4\\DO3"(w516, error in=w518) -> (error out=w517:errorcluster)
            n238 = shared-variable "RT CompactRIO Target\\Mod3\\DI13"(error in=w517) -> (w534:bool, error out=w509:errorcluster)
            n239 = Get Queue Status(queue=w510, error in (no error)=w509) -> (queue out=w505:refnum<queue>, error out=w504:errorcluster, # elements in queue=w508:i32)  [unwired: 1 in, 5 out]
            n240 = Greater?(x=w508, y=0) -> (0:w506:bool)
            n241 = case shown="False" w506 {
              tunnel: w504 -> [w537 w546]
              tunnel: w505 -> [w536 w545]
              tunnel: [w537 w539] -> w512
              tunnel: [w536 w538] -> w511
              frame False {
              }
              frame True {
                n242 = Preview Queue Element(queue=w545, error in (no error)=w546) -> (queue out=w541:refnum<queue>, element=w544:string, error out=w540:errorcluster)  [unwired: 1 in, 1 out]
                n243 = Equal?(x=w544, y="Shutdown") -> (x = y?=w542:bool)
                n244 = case shown="True" w542 {
                  tunnel: w541 -> [w548 w553]
                  tunnel: w540 -> [w547 w552]
                  tunnel: [w547 w551] -> w539
                  tunnel: [w548 w549] -> w538
                  frame False {
                  }
                  frame True {
                    n245 = local write "SDFlag"(TRUE ("SDFlag")) -> ()
                    n246 = Flush Queue(queue=w553, error in (no error)=w552) -> (queue out=w549:refnum<queue>, error out=w551:errorcluster)  [unwired: 1 out]
                  }
                }
              }
            }
            n247 = feedback #7() -> (w514:dbl)  [unwired: 1 in]
            n248 = case shown="True" w534 {
              tunnel: [w561 w607] -> w535
              tunnel: w512 -> [w562 w605]
              tunnel: w511 -> [w557 w600]
              tunnel: [w555 0.0] -> w513
              tunnel: w514 -> [w554 _]
              frame False {
                n249 = call "Regular Timer Action Engine.vi"("Enum"=Control_Timer."Timecheck", "Time Target"=0.5, "error in"=w562) -> ("Status"=w566:cluster{"Running":bool, "Done":bool}, "error out"=w563:errorcluster)  [unwired: 6 in]
                n250 = Unbundle By Name(w566) -> ("Done"=w565:bool)  [unwired: 1 out]
                n251 = feedback #8() -> (w564:bool)  [unwired: 1 in]
                n252 = case shown="False" w565 {
                  tunnel: [w573 w586] -> w558
                  tunnel: w564 -> [w573 w585]
                  tunnel: w563 -> [w572 w577]
                  tunnel: [w572 w583] -> w560
                  tunnel: w557 -> [w571 w579]
                  tunnel: [w571 w578] -> w556
                  tunnel: [w570 w575] -> w555
                  tunnel: w554 -> [w570 w574]
                  frame False {
                  }
                  frame True {
                    n253 = Increment(x=w574) -> (x+1=w580:dbl)
                    n254 = local write "BrojacGreska"(w580) -> ()
                    n255 = Greater Or Equal?(x=w580, y=29.0) -> (x >= y?=w581:bool)
                    n256 = case shown="True" w581 {
                      tunnel: [w589 0.0] -> w575
                      tunnel: w580 -> [w589 _]
                      tunnel: w579 -> [w587 w591]
                      tunnel: [w587 w593] -> w578
                      tunnel: w577 -> [w588 w590]
                      tunnel: [w588 w592] -> w576
                      frame False {
                      }
                      frame True {
                        n257 = Enqueue Element At Opposite End(queue=w591, element="EmergencyOff", error in (no error)=w590) -> (queue out=w593:refnum<queue>, error out=w592:errorcluster)  [unwired: 1 in, 1 out]
                      }
                    }
                    n258 = Not(x=w585) -> (.not. x?=w586:bool)
                    n259 = call "Regular Timer Action Engine.vi"("Enum"=Control_Timer."Reset", "error in"=w576) -> ("error out"=w583:errorcluster)  [unwired: 7 in, 1 out]
                  }
                }
                n260 = feedback-in #8(w558) -> ()
                n261 = local write "CenterLED"(w558) -> ()
                n262 = shared-variable "RT CompactRIO Target\\Mod4\\DO2"(w558, error in=w560) -> (error out=w559:errorcluster)
                n263 = Enqueue Element(queue=w556, element="MoveCenter", error in (no error)=w559) -> (error out=w561:errorcluster)  [unwired: 1 in, 2 out]
              }
              frame True {
                w601 = TRUE ("DO2")
                # "DODATA OBRADA PUMP FLAGA AKO NIJE SD FLAG"
                n264 = shared-variable "RT CompactRIO Target\\Mod4\\DO13"(FALSE ("DO15"), error in=w605) -> (error out=w604:errorcluster)
                n265 = shared-variable "RT CompactRIO Target\\Mod4\\DO12"(FALSE ("DO14"), error in=w604) -> (error out=w603:errorcluster)
                n266 = local write "CenterLED"(w601) -> ()
                n267 = shared-variable "RT CompactRIO Target\\Mod4\\DO2"(w601, error in=w603) -> (error out=w602:errorcluster)
                n268 = local read "SDFlag"() -> (w597:bool)
                n269 = local read "PumpFlag"() -> (w596:bool)
                n270 = case shown="True" w597 {
                  tunnel: [w611 w623] -> w607
                  tunnel: w602 -> [w610 w625]
                  tunnel: w600 -> [w609 w624]
                  tunnel: w596 -> [w608 _]
                  frame False {
                    n271 = case shown="False" w608 {
                      tunnel: [w614 w618] -> w611
                      tunnel: w610 -> [w613 w620]
                      tunnel: w609 -> [w612 w619]
                      frame False {
                        n272 = Enqueue Element(queue=w612, element="Ready", error in (no error)=w613) -> (error out=w614:errorcluster)  [unwired: 1 in, 2 out]
                      }
                      frame True {
                        n273 = local write "PumpFlag"(FALSE ("PumpFlag")) -> ()
                        n274 = Enqueue Element(queue=w619, element="Pump", error in (no error)=w620) -> (error out=w618:errorcluster)  [unwired: 1 in, 2 out]
                      }
                    }
                  }
                  frame True {
                    n275 = local write "SDFlag"(FALSE ("SDFlag")) -> ()
                    n276 = Enqueue Element(queue=w624, element="Shutdown", error in (no error)=w625) -> (error out=w623:errorcluster)  [unwired: 1 in, 2 out]
                  }
                }
              }
            }
            n277 = feedback-in #7(w513) -> ()
          }
          frame True {
            # "DODAT FALG UMESTO POKRETANJA PUMPE ODMAH"
            n278 = local write "PumpFlag"(TRUE ("PumpFlag")) -> ()
            n279 = Enqueue Element(queue=w627, element="MoveCenter", error in (no error)=w629) -> (error out=w628:errorcluster)  [unwired: 1 in, 2 out]
          }
        }
      }
      frame "Ready" {
        n280 = shared-variable "RT CompactRIO Target\\Mod3\\DI6"(error in=w634) -> (w633:bool, error out=w631:errorcluster)
        n281 = call <vilib>:"Boolean Crossing PtByPt.vi"("direction"=enum16{"either", "false-true", "true-false"}."false-true", "input"=w633) -> ("crossing"=w632:bool)  [unwired: 1 in]
        n282 = case shown="False" w632 {
          tunnel: [w639 w681] -> w638
          tunnel: w637 -> [w646 _]
          tunnel: w636 -> [w645 w680]
          tunnel: w631 -> [w640 w678]
          frame False {
            n283 = Get Queue Status(queue=w645) -> (queue out=w644:refnum<queue>, # elements in queue=w642:i32)  [unwired: 2 in, 6 out]
            n284 = Greater?(x=w642, y=0) -> (0:w643:bool)
            n285 = case shown="False" w643 {
              tunnel: [w647 w667] -> w639
              tunnel: w646 -> [w649 w666]
              tunnel: w644 -> [w650 w657]
              tunnel: w640 -> [w648 w656]
              frame False {
                n286 = Enqueue Element(queue=w650, element=w649, error in (no error)=w648) -> (error out=w647:errorcluster)  [unwired: 1 in, 2 out]
              }
              frame True {
                n287 = Preview Queue Element(queue=w657, error in (no error)=w656) -> (queue out=w653:refnum<queue>, element=w655:string, error out=w652:errorcluster)  [unwired: 1 in, 1 out]
                n288 = Equal?(x=w655, y="MoveRight") -> (x = y?=w662:bool)
                n289 = Equal?(x=w655, y="MoveLeft") -> (x = y?=w661:bool)
                n290 = Equal?(x=w655, y="MoveCenter") -> (x = y?=w659:bool)
                n291 = Equal?(x=w655, y="Shutdown") -> (x = y?=w651:bool)
                n292 = Or(x=w662, y=w661) -> (x .or. y?=w660:bool)
                n293 = Or(x=w660, y=w659) -> (x .or. y?=w658:bool)
                n294 = case shown="False" w658 {
                  tunnel: [w668 w677] -> w667
                  tunnel: w666 -> [_ _]
                  tunnel: w653 -> [w670 _]
                  tunnel: w652 -> [w669 w677]
                  tunnel: w651 -> [w671 _]
                  frame False {
                    n295 = case shown="False" w671 {
                      tunnel: w670 -> [w674 _]
                      tunnel: w669 -> [w673 w676]
                      tunnel: [w672 w676] -> w668
                      frame False {
                        n296 = Enqueue Element(queue=w674, element="Ready", error in (no error)=w673) -> (error out=w672:errorcluster)  [unwired: 1 in, 2 out]
                      }
                      frame True {
                      }
                    }
                  }
                  frame True {
                  }
                }
              }
            }
          }
          frame True {
            n297 = Enqueue Element(queue=w680, element="Pump", error in (no error)=w678) -> (error out=w681:errorcluster)  [unwired: 1 in, 2 out]
          }
        }
      }
    }
  }
  n298 = while {
    tunnel: w9 -> [w698]
    tunnel: [w695] -> w7
    shift-right: [w693] -> w5
    shift-left: w2 -> [w692]
    stop <- FALSE stop-if-true
    n299 = event shown="[7] \"RightAct\": Value Change" {
      selector: _ -> [_ _ _ _ _ _ _ _ _ _ _ _]
      dyn-events: _ -> [_ _ _ _ _ _ _ _ _ _ _ _]
      timeout: _ -> [_ _ _ _ _ _ _ _ _ _ _ _]
      tunnel: w698 -> [w700 w747 w798 w805 w811 w832 w855 w891 w927 w963 w999 w1051]
      tunnel: [w705 w752 w797 w804 w810 w831 w857 w893 w929 w965 w1001 w1053] -> w697
      tunnel: [w704 w751 w796 w803 w809 w830 w856 w892 w928 w964 w1000 w1052] -> w696
      tunnel: w692 -> [w699 w746 w793 w800 w807 w829 w849 w885 w921 w957 w993 w1045]
      event "On": Value Change {
        n300 = event-data() -> ()  [unwired: 1 in, 6 out]
        n301 = local read "Stanje"() -> (w701:string)
        n302 = Equal?(x=w701, y="Init") -> (x = y?=w702:bool)
        n303 = case shown="True" w702 {
          tunnel: [w706 w723] -> w705
          tunnel: [w707 w722] -> w704
          tunnel: w700 -> [w707 w709]
          tunnel: w699 -> [w706 w708]
          frame False {
          }
          frame True {
            w710 = TRUE
            n304 = shared-variable "RT CompactRIO Target\\Mod3\\DI8"(error in=w708) -> (w716:bool, error out=w713:errorcluster)
            n305 = shared-variable "RT CompactRIO Target\\Mod3\\DI10"(error in=w713) -> (w717:bool, error out=w712:errorcluster)
            n306 = shared-variable "RT CompactRIO Target\\Mod3\\DI12"(error in=w712) -> (w718:bool, error out=w711:errorcluster)
            n307 = Build Array(w716, w717, w718) -> (w715:bool[])
            n308 = And Array Elements(Boolean array=w715) -> (logical AND=w714:bool)
            n309 = shared-variable "RT CompactRIO Target\\Mod4\\DO0"(w710, error in=w711) -> (error out=w719:errorcluster)
            n310 = local write "On/Off"(w710) -> ()
            n311 = shared-variable "RT CompactRIO Target\\Mod3\\DI6"(error in=w719) -> (w721:bool, error out=w720:errorcluster)
            n312 = case shown="False" w721 {
              tunnel: [w728 w744] -> w723
              tunnel: [w727 w743] -> w722
              tunnel: w720 -> [w726 w742]
              tunnel: w714 -> [w725 _]
              tunnel: w709 -> [w724 w741]
              frame False {
                n313 = case shown="False" w725 {
                  tunnel: [w734 w740] -> w728
                  tunnel: [w733 w738] -> w727
                  tunnel: w726 -> [w735 w737]
                  tunnel: w724 -> [w731 w736]
                  frame False {
                    # "DODATO POKRETANJE MOTORA"
                    n314 = shared-variable "RT CompactRIO Target\\Mod4\\DO11"(TRUE ("DO11")) -> ()  [unwired: 1 in, 1 out]
                    n315 = shared-variable "RT CompactRIO Target\\Mod4\\DO13"(TRUE ("DO13")) -> ()  [unwired: 1 in, 1 out]
                    n316 = Enqueue Element(queue=w731, element="MoveLeft", error in (no error)=w735) -> (queue out=w733:refnum<queue>, error out=w734:errorcluster)  [unwired: 1 in, 1 out]
                  }
                  frame True {
                    n317 = Enqueue Element(queue=w736, element="Ready", error in (no error)=w737) -> (queue out=w738:refnum<queue>, error out=w740:errorcluster)  [unwired: 1 in, 1 out]
                  }
                }
              }
              frame True {
                n318 = Enqueue Element(queue=w741, element="Pump", error in (no error)=w742) -> (queue out=w743:refnum<queue>, error out=w744:errorcluster)  [unwired: 1 in, 1 out]
              }
            }
          }
        }
      }
      event "OnAct": Value Change {
        n319 = event-data() -> ()  [unwired: 1 in, 6 out]
        n320 = invoke on="OnAct" class="Bool (strict)" method="Reinit To Default"() -> ()  [unwired: 3 in, 3 out]
        n321 = local read "Stanje"() -> (w748:string)
        n322 = Equal?(x=w748, y="Init") -> (x = y?=w749:bool)
        n323 = case shown="True" w749 {
          tunnel: [w753 w770] -> w752
          tunnel: [w754 w769] -> w751
          tunnel: w747 -> [w754 w756]
          tunnel: w746 -> [w753 w755]
          frame False {
          }
          frame True {
            w757 = TRUE
            n324 = shared-variable "RT CompactRIO Target\\Mod3\\DI8"(error in=w755) -> (w763:bool, error out=w760:errorcluster)
            n325 = shared-variable "RT CompactRIO Target\\Mod3\\DI10"(error in=w760) -> (w764:bool, error out=w759:errorcluster)
            n326 = shared-variable "RT CompactRIO Target\\Mod3\\DI12"(error in=w759) -> (w765:bool, error out=w758:errorcluster)
            n327 = Build Array(w763, w764, w765) -> (w762:bool[])
            n328 = And Array Elements(Boolean array=w762) -> (logical AND=w761:bool)
            n329 = shared-variable "RT CompactRIO Target\\Mod4\\DO0"(w757, error in=w758) -> (error out=w766:errorcluster)
            n330 = local write "On/Off"(w757) -> ()
            n331 = shared-variable "RT CompactRIO Target\\Mod3\\DI6"(error in=w766) -> (w768:bool, error out=w767:errorcluster)
            n332 = case shown="False" w768 {
              tunnel: [w775 w791] -> w770
              tunnel: [w774 w790] -> w769
              tunnel: w767 -> [w773 w789]
              tunnel: w761 -> [w772 _]
              tunnel: w756 -> [w771 w788]
              frame False {
                n333 = case shown="False" w772 {
                  tunnel: [w781 w787] -> w775
                  tunnel: [w780 w785] -> w774
                  tunnel: w773 -> [w782 w784]
                  tunnel: w771 -> [w778 w783]
                  frame False {
                    # "DODATO POKRETANJE MOTORA"
                    n334 = shared-variable "RT CompactRIO Target\\Mod4\\DO11"(TRUE ("DO11")) -> ()  [unwired: 1 in, 1 out]
                    n335 = shared-variable "RT CompactRIO Target\\Mod4\\DO13"(TRUE ("DO13")) -> ()  [unwired: 1 in, 1 out]
                    n336 = Enqueue Element(queue=w778, element="MoveLeft", error in (no error)=w782) -> (queue out=w780:refnum<queue>, error out=w781:errorcluster)  [unwired: 1 in, 1 out]
                  }
                  frame True {
                    n337 = Enqueue Element(queue=w783, element="Ready", error in (no error)=w784) -> (queue out=w785:refnum<queue>, error out=w787:errorcluster)  [unwired: 1 in, 1 out]
                  }
                }
              }
              frame True {
                n338 = Enqueue Element(queue=w788, element="Pump", error in (no error)=w789) -> (queue out=w790:refnum<queue>, error out=w791:errorcluster)  [unwired: 1 in, 1 out]
              }
            }
          }
        }
      }
      event "Off": Value Change {
        w794 = FALSE
        n339 = event-data() -> ()  [unwired: 1 in, 6 out]
        n340 = shared-variable "RT CompactRIO Target\\Mod4\\DO0"(w794, error in=w793) -> (error out=w795:errorcluster)
        n341 = local write "On/Off"(w794) -> ()
        n342 = Enqueue Element(queue=w798, element="Shutdown", error in (no error)=w795) -> (queue out=w796:refnum<queue>, error out=w797:errorcluster)  [unwired: 1 in, 1 out]
      }
      event "OffAct": Value Change {
        w801 = FALSE
        n343 = event-data() -> ()  [unwired: 1 in, 6 out]
        n344 = invoke on="OffAct" class="Bool (strict)" method="Reinit To Default"() -> ()  [unwired: 3 in, 3 out]
        n345 = shared-variable "RT CompactRIO Target\\Mod4\\DO0"(w801, error in=w800) -> (error out=w802:errorcluster)
        n346 = local write "On/Off"(w801) -> ()
        n347 = Enqueue Element(queue=w805, element="Shutdown", error in (no error)=w802) -> (queue out=w803:refnum<queue>, error out=w804:errorcluster)  [unwired: 1 in, 1 out]
      }
      event "Emergency off": Value Change {
        # "PROMENJENO FALSE U TRUE  ZBOG OBRNUTE LOGIKE OFFA"
        n348 = event-data() -> ()  [unwired: 1 in, 6 out]
        n349 = case shown="False" "Emergency off" {
          tunnel: w811 -> [w817 w827]
          tunnel: [w816 w826] -> w810
          tunnel: [w815 w825] -> w809
          tunnel: w807 -> [w813 w819]
          frame False {
            w812 = TRUE ("DO4")
            w814 = FALSE
            n350 = shared-variable "RT CompactRIO Target\\Mod4\\DO0"(w814) -> ()  [unwired: 1 in, 1 out]
            n351 = local write "On/Off"(w814) -> ()
            n352 = local write "Fault"(w812) -> ()
            n353 = shared-variable "RT CompactRIO Target\\Mod4\\DO4"(w812) -> ()  [unwired: 1 in, 1 out]
            n354 = Enqueue Element At Opposite End(queue=w817, element="EmergencyOff", error in (no error)=w813) -> (queue out=w815:refnum<queue>, error out=w816:errorcluster)  [unwired: 1 in, 1 out]
          }
          frame True {
            n355 = Flush Queue(queue=w827, error in (no error)=w819) -> (queue out=w824:refnum<queue>, error out=w821:errorcluster)  [unwired: 1 out]
            n356 = shared-variable "RT CompactRIO Target\\Mod4\\DO4"(FALSE ("DO4"), error in=w821) -> (error out=w820:errorcluster)
            n357 = Enqueue Element(queue=w824, element="Init", error in (no error)=w820) -> (queue out=w825:refnum<queue>, error out=w826:errorcluster)  [unwired: 1 in, 1 out]
          }
        }
      }
      event "Emergency offAct": Value Change {
        # "PROMENJENO FALSE U TRUE  ZBOG OBRNUTE LOGIKE OFFA"
        n358 = event-data() -> ()  [unwired: 1 in, 6 out]
        n359 = case shown="True" "Emergency offAct" {
          tunnel: w832 -> [w838 w848]
          tunnel: [w837 w847] -> w831
          tunnel: [w836 w846] -> w830
          tunnel: w829 -> [w834 w840]
          frame False {
            w833 = TRUE ("DO4")
            w835 = FALSE
            n360 = shared-variable "RT CompactRIO Target\\Mod4\\DO0"(w835) -> ()  [unwired: 1 in, 1 out]
            n361 = local write "On/Off"(w835) -> ()
            n362 = local write "Fault"(w833) -> ()
            n363 = shared-variable "RT CompactRIO Target\\Mod4\\DO4"(w833) -> ()  [unwired: 1 in, 1 out]
            n364 = Enqueue Element At Opposite End(queue=w838, element="EmergencyOff", error in (no error)=w834) -> (queue out=w836:refnum<queue>, error out=w837:errorcluster)  [unwired: 1 in, 1 out]
          }
          frame True {
            n365 = Flush Queue(queue=w848, error in (no error)=w840) -> (queue out=w845:refnum<queue>, error out=w842:errorcluster)  [unwired: 1 out]
            n366 = shared-variable "RT CompactRIO Target\\Mod4\\DO4"(FALSE ("DO4"), error in=w842) -> (error out=w841:errorcluster)
            n367 = Enqueue Element(queue=w845, element="Init", error in (no error)=w841) -> (queue out=w846:refnum<queue>, error out=w847:errorcluster)  [unwired: 1 in, 1 out]
          }
        }
      }
      event "Right": Value Change {
        n368 = event-data() -> ()  [unwired: 1 in, 6 out]
        n369 = local read "Stanje"() -> (w854:string)
        n370 = call "Regular Timer Action Engine.vi"("Enum"=Control_Timer."Reset", "error in"=w849) -> ("error out"=w850:errorcluster)  [unwired: 7 in, 1 out]
        n371 = Equal?(x=w854, y="Ready") -> (x = y?=w852:bool)
        n372 = case shown="True" w852 {
          tunnel: w850 -> [w859 w867]
          tunnel: [w859 w864] -> w857
          tunnel: [w858 w863] -> w856
          tunnel: w855 -> [w858 w862]
          frame False {
          }
          frame True {
            n373 = shared-variable "RT CompactRIO Target\\Mod3\\DI9"(error in=w867) -> (w869:bool, error out=w866:errorcluster)
            n374 = shared-variable "RT CompactRIO Target\\Mod3\\DI11"(error in=w866) -> (w870:bool, error out=w865:errorcluster)
            n375 = shared-variable "RT CompactRIO Target\\Mod3\\DI14"(error in=w865) -> (w871:bool, error out=w860:errorcluster)
            n376 = Build Array(w869, w870, w871) -> (w868:bool[])
            n377 = And Array Elements(Boolean array=w868) -> (logical AND=w861:bool)
            n378 = case shown="False" w861 {
              tunnel: [w881 w883] -> w864
              tunnel: [w880 w884] -> w863
              tunnel: w862 -> [w873 w884]
              tunnel: w860 -> [w872 w883]
              frame False {
                n379 = shared-variable "RT CompactRIO Target\\Mod4\\DO12"(TRUE ("DO15"), error in=w872) -> (error out=w876:errorcluster)
                n380 = shared-variable "RT CompactRIO Target\\Mod4\\DO10"(TRUE ("DO13"), error in=w876) -> (error out=w875:errorcluster)
                n381 = shared-variable "RT CompactRIO Target\\Mod4\\DO9"(TRUE ("DO11"), error in=w875) -> (error out=w874:errorcluster)
                n382 = Enqueue Element(queue=w873, element="MoveRight", error in (no error)=w874) -> (queue out=w880:refnum<queue>, error out=w881:errorcluster)  [unwired: 1 in, 1 out]
              }
              frame True {
              }
            }
          }
        }
      }
      event "RightAct": Value Change {
        n383 = event-data() -> ()  [unwired: 1 in, 6 out]
        n384 = invoke on="RightAct" class="Bool (strict)" method="Reinit To Default"() -> ()  [unwired: 3 in, 3 out]
        n385 = local read "Stanje"() -> (w890:string)
        n386 = call "Regular Timer Action Engine.vi"("Enum"=Control_Timer."Reset", "error in"=w885) -> ("error out"=w886:errorcluster)  [unwired: 7 in, 1 out]
        n387 = Equal?(x=w890, y="Ready") -> (x = y?=w888:bool)
        n388 = case shown="True" w888 {
          tunnel: w886 -> [w895 w903]
          tunnel: [w895 w900] -> w893
          tunnel: [w894 w899] -> w892
          tunnel: w891 -> [w894 w898]
          frame False {
          }
          frame True {
            n389 = shared-variable "RT CompactRIO Target\\Mod3\\DI9"(error in=w903) -> (w905:bool, error out=w902:errorcluster)
            n390 = shared-variable "RT CompactRIO Target\\Mod3\\DI11"(error in=w902) -> (w906:bool, error out=w901:errorcluster)
            n391 = shared-variable "RT CompactRIO Target\\Mod3\\DI14"(error in=w901) -> (w907:bool, error out=w896:errorcluster)
            n392 = Build Array(w905, w906, w907) -> (w904:bool[])
            n393 = And Array Elements(Boolean array=w904) -> (logical AND=w897:bool)
            n394 = case shown="False" w897 {
              tunnel: [w917 w919] -> w900
              tunnel: [w916 w920] -> w899
              tunnel: w898 -> [w909 w920]
              tunnel: w896 -> [w908 w919]
              frame False {
                n395 = shared-variable "RT CompactRIO Target\\Mod4\\DO12"(TRUE ("DO15"), error in=w908) -> (error out=w912:errorcluster)
                n396 = shared-variable "RT CompactRIO Target\\Mod4\\DO10"(TRUE ("DO13"), error in=w912) -> (error out=w911:errorcluster)
                n397 = shared-variable "RT CompactRIO Target\\Mod4\\DO9"(TRUE ("DO11"), error in=w911) -> (error out=w910:errorcluster)
                n398 = Enqueue Element(queue=w909, element="MoveRight", error in (no error)=w910) -> (queue out=w916:refnum<queue>, error out=w917:errorcluster)  [unwired: 1 in, 1 out]
              }
              frame True {
              }
            }
          }
        }
      }
      event "Left": Value Change {
        n399 = event-data() -> ()  [unwired: 1 in, 6 out]
        n400 = local read "Stanje"() -> (w926:string)
        n401 = call "Regular Timer Action Engine.vi"("Enum"=Control_Timer."Reset", "error in"=w921) -> ("error out"=w922:errorcluster)  [unwired: 7 in, 1 out]
        n402 = Equal?(x=w926, y="Ready") -> (x = y?=w924:bool)
        n403 = case shown="True" w924 {
          tunnel: w922 -> [w931 w939]
          tunnel: [w931 w936] -> w929
          tunnel: [w930 w935] -> w928
          tunnel: w927 -> [w930 w934]
          frame False {
          }
          frame True {
            n404 = shared-variable "RT CompactRIO Target\\Mod3\\DI8"(error in=w939) -> (w941:bool, error out=w938:errorcluster)
            n405 = shared-variable "RT CompactRIO Target\\Mod3\\DI10"(error in=w938) -> (w942:bool, error out=w937:errorcluster)
            n406 = shared-variable "RT CompactRIO Target\\Mod3\\DI12"(error in=w937) -> (w943:bool, error out=w932:errorcluster)
            n407 = Build Array(w941, w942, w943) -> (w940:bool[])
            n408 = And Array Elements(Boolean array=w940) -> (logical AND=w933:bool)
            n409 = case shown="False" w933 {
              tunnel: [w953 w955] -> w936
              tunnel: [w951 w956] -> w935
              tunnel: w934 -> [w952 w956]
              tunnel: w932 -> [w944 w955]
              frame False {
                n410 = shared-variable "RT CompactRIO Target\\Mod4\\DO13"(TRUE ("DO15"), error in=w944) -> (error out=w948:errorcluster)
                n411 = shared-variable "RT CompactRIO Target\\Mod4\\DO11"(TRUE ("DO13"), error in=w948) -> (error out=w947:errorcluster)
                n412 = shared-variable "RT CompactRIO Target\\Mod4\\DO9"(FALSE ("DO9"), error in=w947) -> (error out=w946:errorcluster)
                n413 = Enqueue Element(queue=w952, element="MoveLeft", error in (no error)=w946) -> (queue out=w951:refnum<queue>, error out=w953:errorcluster)  [unwired: 1 in, 1 out]
              }
              frame True {
              }
            }
          }
        }
      }
      event "LeftAct": Value Change {
        n414 = event-data() -> ()  [unwired: 1 in, 6 out]
        n415 = invoke on="LeftAct" class="Bool (strict)" method="Reinit To Default"() -> ()  [unwired: 3 in, 3 out]
        n416 = local read "Stanje"() -> (w962:string)
        n417 = call "Regular Timer Action Engine.vi"("Enum"=Control_Timer."Reset", "error in"=w957) -> ("error out"=w958:errorcluster)  [unwired: 7 in, 1 out]
        n418 = Equal?(x=w962, y="Ready") -> (x = y?=w960:bool)
        n419 = case shown="True" w960 {
          tunnel: w958 -> [w967 w975]
          tunnel: [w967 w972] -> w965
          tunnel: [w966 w971] -> w964
          tunnel: w963 -> [w966 w970]
          frame False {
          }
          frame True {
            n420 = shared-variable "RT CompactRIO Target\\Mod3\\DI8"(error in=w975) -> (w977:bool, error out=w974:errorcluster)
            n421 = shared-variable "RT CompactRIO Target\\Mod3\\DI10"(error in=w974) -> (w978:bool, error out=w973:errorcluster)
            n422 = shared-variable "RT CompactRIO Target\\Mod3\\DI12"(error in=w973) -> (w979:bool, error out=w969:errorcluster)
            n423 = Build Array(w977, w978, w979) -> (w976:bool[])
            n424 = And Array Elements(Boolean array=w976) -> (logical AND=w968:bool)
            n425 = case shown="True" w968 {
              tunnel: [w989 w991] -> w972
              tunnel: [w987 w992] -> w971
              tunnel: w970 -> [w988 w992]
              tunnel: w969 -> [w980 w991]
              frame False {
                n426 = shared-variable "RT CompactRIO Target\\Mod4\\DO13"(TRUE ("DO15"), error in=w980) -> (error out=w984:errorcluster)
                n427 = shared-variable "RT CompactRIO Target\\Mod4\\DO11"(TRUE ("DO13"), error in=w984) -> (error out=w983:errorcluster)
                n428 = shared-variable "RT CompactRIO Target\\Mod4\\DO9"(FALSE ("DO9"), error in=w983) -> (error out=w982:errorcluster)
                n429 = Enqueue Element(queue=w988, element="MoveLeft", error in (no error)=w982) -> (queue out=w987:refnum<queue>, error out=w989:errorcluster)  [unwired: 1 in, 1 out]
              }
              frame True {
              }
            }
          }
        }
      }
      event "Center": Value Change {
        n430 = event-data() -> ()  [unwired: 1 in, 6 out]
        n431 = local read "Stanje"() -> (w996:string)
        n432 = Equal?(x=w996, y="Ready") -> (x = y?=w997:bool)
        n433 = call "Regular Timer Action Engine.vi"("Enum"=Control_Timer."Reset", "error in"=w993) -> ("error out"=w995:errorcluster)  [unwired: 7 in, 1 out]
        n434 = case shown="True" w997 {
          tunnel: w995 -> [w1003 w1019]
          tunnel: [w1003 w1016] -> w1001
          tunnel: [w1002 w1015] -> w1000
          tunnel: w999 -> [w1002 w1014]
          frame False {
          }
          frame True {
            n435 = shared-variable "RT CompactRIO Target\\Mod3\\DI9"(error in=w1019) -> (w1023:bool, error out=w1018:errorcluster)
            n436 = shared-variable "RT CompactRIO Target\\Mod3\\DI11"(error in=w1018) -> (w1024:bool, error out=w1017:errorcluster)
            n437 = shared-variable "RT CompactRIO Target\\Mod3\\DI14"(error in=w1017) -> (w1004:bool, error out=w1010:errorcluster)
            n438 = shared-variable "RT CompactRIO Target\\Mod3\\DI8"(error in=w1010) -> (w1012:bool, error out=w1009:errorcluster)
            n439 = Build Array(w1023, w1024, w1004) -> (w1022:bool[])
            n440 = shared-variable "RT CompactRIO Target\\Mod3\\DI10"(error in=w1009) -> (w1013:bool, error out=w1008:errorcluster)
            n441 = And Array Elements(Boolean array=w1022) -> (logical AND=w1020:bool)
            n442 = shared-variable "RT CompactRIO Target\\Mod3\\DI12"(error in=w1008) -> (w1005:bool, error out=w1007:errorcluster)
            n443 = Build Array(w1012, w1013, w1005) -> (w1011:bool[])
            n444 = And Array Elements(Boolean array=w1011) -> (logical AND=w1006:bool)
            n445 = Or(x=w1020, y=w1006) -> (x .or. y?=w1021:bool)
            n446 = case shown="True" w1021 {
              tunnel: w1007 -> [w1026 w1028]
              tunnel: [w1026 w1033] -> w1016
              tunnel: [w1025 w1031] -> w1015
              tunnel: w1014 -> [w1025 w1032]
              tunnel: w1005 -> [_ w1030]
              tunnel: w1004 -> [_ w1029]
              frame False {
              }
              frame True {
                n447 = case shown="False" w1030 {
                  tunnel: w1029 -> [w1037 _]
                  tunnel: w1028 -> [w1036 w1043]
                  tunnel: [w1035 w1042] -> w1027
                  frame False {
                    n448 = case shown="False" w1037 {
                      tunnel: w1036 -> [w1038 w1040]
                      tunnel: [w1038 w1039] -> w1035
                      frame False {
                      }
                      frame True {
                        n449 = shared-variable "RT CompactRIO Target\\Mod4\\DO13"(TRUE ("DO15"), error in=w1040) -> (error out=w1039:errorcluster)
                      }
                    }
                  }
                  frame True {
                    n450 = shared-variable "RT CompactRIO Target\\Mod4\\DO12"(TRUE ("DO14"), error in=w1043) -> (error out=w1042:errorcluster)
                  }
                }
                n451 = Enqueue Element(queue=w1032, element="MoveCenter", error in (no error)=w1027) -> (queue out=w1031:refnum<queue>, error out=w1033:errorcluster)  [unwired: 1 in, 1 out]
              }
            }
          }
        }
      }
      event "CenterAct": Value Change {
        n452 = event-data() -> ()  [unwired: 1 in, 6 out]
        n453 = local read "Stanje"() -> (w1048:string)
        n454 = invoke on="CenterAct" class="Bool (strict)" method="Reinit To Default"() -> ()  [unwired: 3 in, 3 out]
        n455 = Equal?(x=w1048, y="Ready") -> (x = y?=w1049:bool)
        n456 = call "Regular Timer Action Engine.vi"("Enum"=Control_Timer."Reset", "error in"=w1045) -> ("error out"=w1047:errorcluster)  [unwired: 7 in, 1 out]
        n457 = case shown="True" w1049 {
          tunnel: w1047 -> [w1055 w1071]
          tunnel: [w1055 w1068] -> w1053
          tunnel: [w1054 w1067] -> w1052
          tunnel: w1051 -> [w1054 w1066]
          frame False {
          }
          frame True {
            n458 = shared-variable "RT CompactRIO Target\\Mod3\\DI9"(error in=w1071) -> (w1075:bool, error out=w1070:errorcluster)
            n459 = shared-variable "RT CompactRIO Target\\Mod3\\DI11"(error in=w1070) -> (w1076:bool, error out=w1069:errorcluster)
            n460 = shared-variable "RT CompactRIO Target\\Mod3\\DI14"(error in=w1069) -> (w1056:bool, error out=w1062:errorcluster)
            n461 = shared-variable "RT CompactRIO Target\\Mod3\\DI8"(error in=w1062) -> (w1064:bool, error out=w1061:errorcluster)
            n462 = Build Array(w1075, w1076, w1056) -> (w1074:bool[])
            n463 = shared-variable "RT CompactRIO Target\\Mod3\\DI10"(error in=w1061) -> (w1065:bool, error out=w1060:errorcluster)
            n464 = And Array Elements(Boolean array=w1074) -> (logical AND=w1072:bool)
            n465 = shared-variable "RT CompactRIO Target\\Mod3\\DI12"(error in=w1060) -> (w1057:bool, error out=w1059:errorcluster)
            n466 = Build Array(w1064, w1065, w1057) -> (w1063:bool[])
            n467 = And Array Elements(Boolean array=w1063) -> (logical AND=w1058:bool)
            n468 = Or(x=w1072, y=w1058) -> (x .or. y?=w1073:bool)
            n469 = case shown="True" w1073 {
              tunnel: w1059 -> [w1078 w1080]
              tunnel: [w1078 w1085] -> w1068
              tunnel: [w1077 w1083] -> w1067
              tunnel: w1066 -> [w1077 w1084]
              tunnel: w1057 -> [_ w1082]
              tunnel: w1056 -> [_ w1081]
              frame False {
              }
              frame True {
                n470 = case shown="False" w1082 {
                  tunnel: w1081 -> [w1089 _]
                  tunnel: w1080 -> [w1088 w1095]
                  tunnel: [w1087 w1094] -> w1079
                  frame False {
                    n471 = case shown="False" w1089 {
                      tunnel: w1088 -> [w1090 w1092]
                      tunnel: [w1090 w1091] -> w1087
                      frame False {
                      }
                      frame True {
                        n472 = shared-variable "RT CompactRIO Target\\Mod4\\DO13"(TRUE ("DO15"), error in=w1092) -> (error out=w1091:errorcluster)
                      }
                    }
                  }
                  frame True {
                    n473 = shared-variable "RT CompactRIO Target\\Mod4\\DO12"(TRUE ("DO14"), error in=w1095) -> (error out=w1094:errorcluster)
                  }
                }
                n474 = Enqueue Element(queue=w1084, element="MoveCenter", error in (no error)=w1079) -> (queue out=w1083:refnum<queue>, error out=w1085:errorcluster)  [unwired: 1 in, 1 out]
              }
            }
          }
        }
      }
    }
    n475 = case shown="No Error" w697 {
      selector: w697 -> [w1097 w1101]
      tunnel: w696 -> [w1098 w1103]
      tunnel: [w1098 w1100] -> w695
      tunnel: [w1097 w1099] -> w693
      frame No Error {
      }
      frame Error {
        n476 = Enqueue Element(queue=w1103, element="Shutdown") -> (queue out=w1100:refnum<queue>, error out=w1102:errorcluster)  [unwired: 2 in, 1 out]
        n477 = Merge Errors(w1102, w1101) -> (w1099:errorcluster)
      }
    }
  }
  n478 = while {
    shift-right: [w1105] -> w1
    shift-left: w2 -> [w1139]
    stop <- FALSE stop-if-true
    n479 = shared-variable "RT CompactRIO Target\\Mod3\\DI0"(error in=w1139) -> (w1137:bool, error out=w1134:errorcluster)
    n480 = shared-variable "RT CompactRIO Target\\Mod3\\DI1"(error in=w1134) -> (w1129:bool, error out=w1133:errorcluster)
    n481 = shared-variable "RT CompactRIO Target\\Mod3\\DI2"(error in=w1133) -> (w1126:bool, error out=w1132:errorcluster)
    n482 = shared-variable "RT CompactRIO Target\\Mod3\\DI3"(error in=w1132) -> (w1123:bool, error out=w1131:errorcluster)
    n483 = shared-variable "RT CompactRIO Target\\Mod3\\DI4"(error in=w1131) -> (w1120:bool, error out=w1130:errorcluster)
    n484 = shared-variable "RT CompactRIO Target\\Mod3\\DI5"(error in=w1130) -> (w1115:bool, error out=w1112:errorcluster)
    n485 = call <vilib>:"Boolean Crossing PtByPt.vi"("direction"=enum16{"either", "false-true", "true-false"}."false-true", "input"=w1137) -> ("crossing"=w1135:bool)  [unwired: 1 in]
    n486 = call <vilib>:"Boolean Crossing PtByPt.vi"("direction"=enum16{"either", "false-true", "true-false"}."true-false", "input"=w1129) -> ("crossing"=w1127:bool)  [unwired: 1 in]
    n487 = call <vilib>:"Boolean Crossing PtByPt.vi"("direction"=enum16{"either", "false-true", "true-false"}."true-false", "input"=w1115) -> ("crossing"=w1117:bool)  [unwired: 1 in]
    n488 = call <vilib>:"Boolean Crossing PtByPt.vi"("direction"=enum16{"either", "false-true", "true-false"}."false-true", "input"=w1126) -> ("crossing"=w1124:bool)  [unwired: 1 in]
    n489 = call <vilib>:"Boolean Crossing PtByPt.vi"("direction"=enum16{"either", "false-true", "true-false"}."false-true", "input"=w1115) -> ("crossing"=w1113:bool)  [unwired: 1 in]
    n490 = call <vilib>:"Boolean Crossing PtByPt.vi"("direction"=enum16{"either", "false-true", "true-false"}."false-true", "input"=w1123) -> ("crossing"=w1121:bool)  [unwired: 1 in]
    n491 = call <vilib>:"Boolean Crossing PtByPt.vi"("direction"=enum16{"either", "false-true", "true-false"}."false-true", "input"=w1120) -> ("crossing"=w1118:bool)  [unwired: 1 in]
    n492 = case shown="True" w1113 {
      tunnel: w1112 -> [w1140 w1142]
      tunnel: [w1140 w1141] -> w1111
      frame False {
      }
      frame True {
        w1143 = TRUE ("Emergency offAct")
        n493 = local write "Emergency offAct"(w1143) -> ()
        n494 = property on="Emergency offAct" class="Bool (strict)"(error in=w1142, "Val(Sgnl)"=w1143) -> (error out=w1141:errorcluster)  [unwired: 1 in, 1 out]
      }
    }
    n495 = case shown="True" w1117 {
      tunnel: w1111 -> [w1144 w1146]
      tunnel: [w1144 w1145] -> w1110
      frame False {
      }
      frame True {
        w1147 = FALSE ("Emergency offAct")
        n496 = local write "Emergency offAct"(w1147) -> ()
        n497 = property on="Emergency offAct" class="Bool (strict)"(error in=w1146, "Val(Sgnl)"=w1147) -> (error out=w1145:errorcluster)  [unwired: 1 in, 1 out]
      }
    }
    n498 = case shown="True" w1118 {
      tunnel: w1110 -> [w1148 w1150]
      tunnel: [w1148 w1149] -> w1109
      frame False {
      }
      frame True {
        w1151 = TRUE ("RightAct")
        n499 = property on="RightAct" class="Bool (strict)"(error in=w1150, "Val(Sgnl)"=w1151) -> (error out=w1149:errorcluster)  [unwired: 1 in, 1 out]
        n500 = local write "RightAct"(w1151) -> ()
      }
    }
    n501 = case shown="True" w1121 {
      tunnel: w1109 -> [w1152 w1154]
      tunnel: [w1152 w1153] -> w1108
      frame False {
      }
      frame True {
        w1155 = TRUE ("CenterAct")
        n502 = local write "CenterAct"(w1155) -> ()
        n503 = property on="CenterAct" class="Bool (strict)"(error in=w1154, "Val(Sgnl)"=w1155) -> (error out=w1153:errorcluster)  [unwired: 1 in, 1 out]
      }
    }
    n504 = case shown="True" w1124 {
      tunnel: w1108 -> [w1156 w1158]
      tunnel: [w1156 w1157] -> w1107
      frame False {
      }
      frame True {
        w1159 = TRUE ("LeftAct")
        n505 = local write "LeftAct"(w1159) -> ()
        n506 = property on="LeftAct" class="Bool (strict)"(error in=w1158, "Val(Sgnl)"=w1159) -> (error out=w1157:errorcluster)  [unwired: 1 in, 1 out]
      }
    }
    n507 = case shown="True" w1127 {
      tunnel: w1107 -> [w1160 w1162]
      tunnel: [w1160 w1161] -> w1106
      frame False {
      }
      frame True {
        w1163 = TRUE ("OffAct")
        n508 = local write "OffAct"(w1163) -> ()
        n509 = property on="OffAct" class="Bool (strict)"(error in=w1162, "Val(Sgnl)"=w1163) -> (error out=w1161:errorcluster)  [unwired: 1 in, 1 out]
      }
    }
    n510 = case shown="True" w1135 {
      tunnel: w1106 -> [w1164 w1166]
      tunnel: [w1164 w1165] -> w1105
      frame False {
      }
      frame True {
        w1167 = TRUE ("On")
        n511 = local write "OnAct"(w1167) -> ()
        n512 = property on="OnAct" class="Bool (strict)"(error in=w1166, "Val(Sgnl)"=w1167) -> (error out=w1165:errorcluster)  [unwired: 1 in, 1 out]
      }
    }
  }
  n513 = Merge Errors(w5, w6, w1) -> (w4:errorcluster)
  n514 = Release Queue(queue=w7, error in (no error)=w4) -> (error out=→"error out":errorcluster)  [unwired: 1 in, 2 out]
